vi "main_machine_no_dilution.vi"() -> ()   [LabVIEW 2013]
uses:
  type_defs/robotics_states.ctl
  type_defs/fsc_parameter.ctl
  type_defs/hts_message.ctl
  type_defs/led_mm.ctl
  type_defs/data_message.ctl
  type_defs/reactor.ctl
  type_defs/experiment_states.ctl
  type_defs/global_settings.ctl
  type_defs/mm_states.ctl
  type_defs/experiment_settings.ctl
  type_defs/ps_states.ctl
  hts/type_defs/hts_command_list.ctl
  <vilib>/Utility/file.llb/Write To Spreadsheet File (DBL).vi
  <vilib>/Utility/file.llb/Read From Spreadsheet File (DBL).vi
panel:
  out "GLOBAL STATE":T1
  out "DILUTION  TABLE":dbl[][](array[numeric])
  in  "SETTINGS":T2={"# REACTORS"=8, "17X PORT"=8, "WASTE POSITION "=3, "SECONDS BETWEEN SAMPLING"=600.0, "FACS DIVA DIRECTORY"=path "D:/BDDatabase/BDData", "DATA FILE"=path "C:/Documents and Settings/HES/Desktop/THN20190207_datafile.csv", "REACTORS TO USE"=[5, 4, 7, 6, 11, 12, 2, 1], "PULSE PERIOD"=60, "USE LIGHTS?"=FALSE, "LED FILE"=path "C:/Documents and Settings/HES/Desktop/THN20190207_lightfile.csv", "LED CHANNELS"=[5, 7, 8, 6, 2, 1, 4, 9], "PULSE LENGTH"=60, "SUMMARY FILE"=path "C:/Documents and Settings/HES/Desktop/THN20190207_summaryfile.csv", "OUTGROWTH TIME POINTS"=1.0, "SELECTION VALVE PORT"="COM4", "HTS PORT"="COM6", "DILUTION VOLUME (uL)"=2000, "DILUTION FILE"=path "C:/Documents and Settings/HES/Desktop/THN20190207_dilutionfile.csv", "1X PORT"=10}
  out "EXPERIMENT STATE":T3
  out "TIME TILL SAMPLE":dbl
  out "TIME POINT":i32
  out "SAMPLE #":i32
  out "ITERATION":u32
  out "REACTOR":T5
  out "mAs":dbl[](array[numeric])
  out "NEXT LIGHTS":bool[](array[boolean])
  out "DATA THREAD":T6
  out "LED THREAD":T7
  out "HTS THREAD":T8=enum."DILUTE AND INDUCE"
  out "TIME TILL STROBE":dbl
  in  "Y":T9 items=["DSRED"=30, "TIME"=0, "FSC"=1, "SSC"=6, "FITC"=9]
  in  "X":T9 items=["DSRED"=30, "TIME"=0, "FSC"=1, "SSC"=6, "FITC"=9]
  in  "Reactor to Graph":i32
  out "LOG FITC/SSC":dbl[](graph)
  out "LOG (X/Y)":dynamicdata(graph) caption="Histogram"
  out "Y VERSUS X":T10(graph)
  in  "GRAPH DATA":bool
  in  "REACTOR #":i32
  in  "SHOW REACTOR":bool
  out "CURRENT VALVE":u32
  out "?":timestamp
  out "?":path
  in  "UPDATE STATES":bool
  out "ROBOTICS READY?":T11
  in  "PAUSE":bool
  in  "START EXPERIMENT":bool
  in  "FIND FCS FILE":bool
  in  "INITIALIZE INSTRUMENT":bool
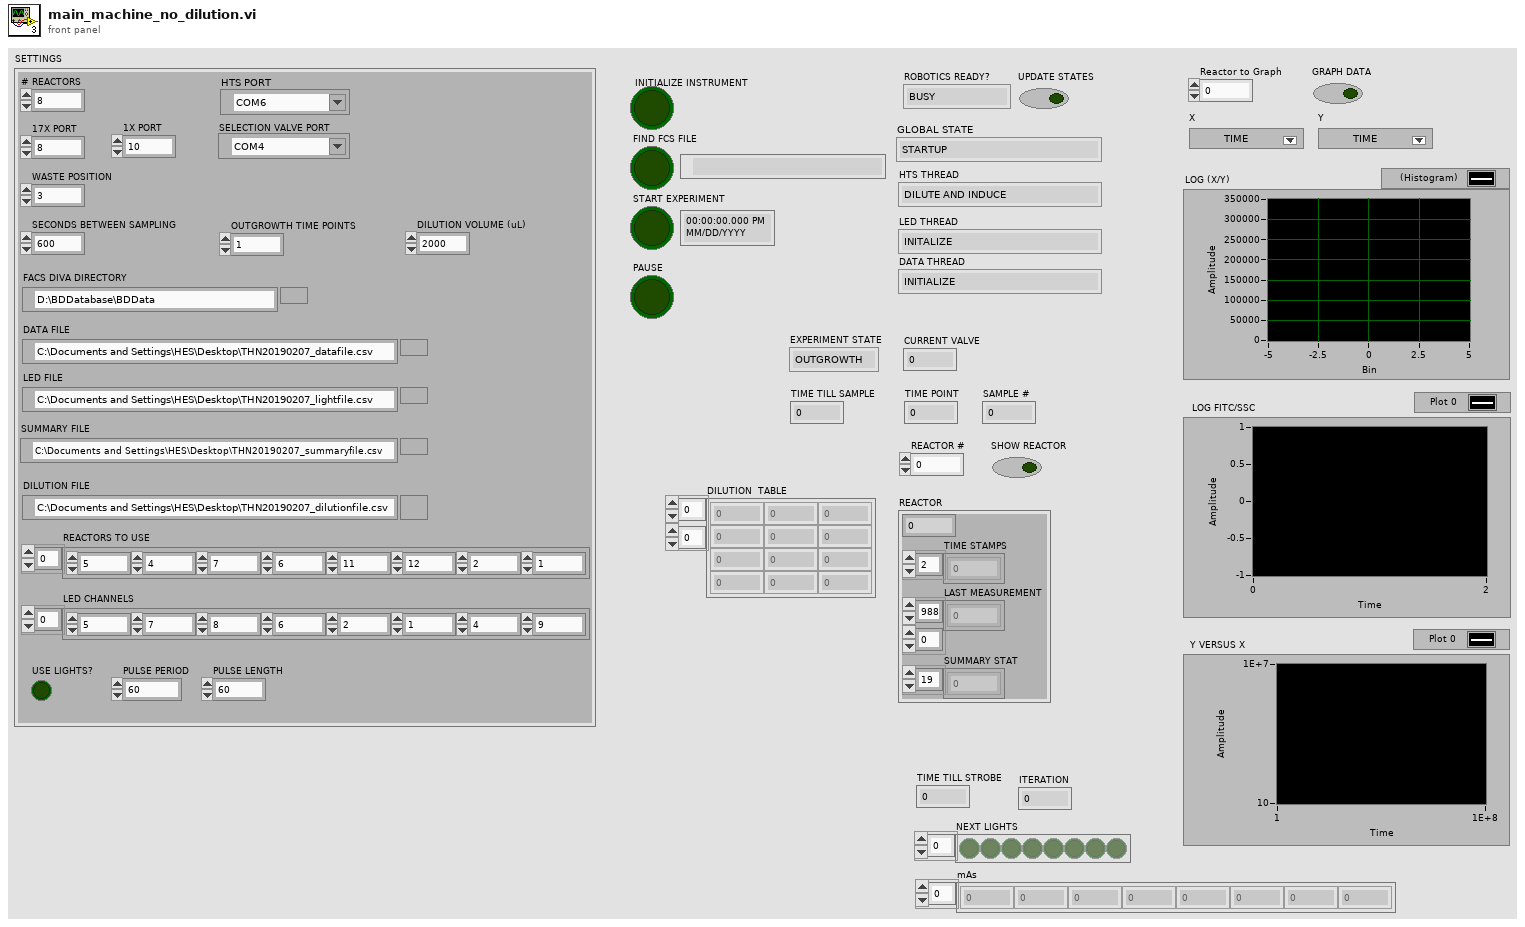
[diagram p1: front panel]
types:
  T1 = typedef "mm_states.ctl" = enum16{"STARTUP", "WAIT FOR COMMAND", "INITIALIZE INSTRUMENT", "FIND FCS FILE ", "START EXPERIMENT", "WAIT TO SAMPLE ", "DILUTE", "TAKE SAMPLE ", "EXIT"}
  T2 = typedef "global_settings.ctl" = cluster{"# REACTORS":u32, "17X PORT":i32, "WASTE POSITION ":i32, "SECONDS BETWEEN SAMPLING":dbl, "FACS DIVA DIRECTORY":path, "DATA FILE":path, "REACTORS TO USE":u32[], "PULSE PERIOD":i32, "USE LIGHTS?":bool, "LED FILE":path, "LED CHANNELS":u32[], "PULSE LENGTH":i32, "SUMMARY FILE":path, "OUTGROWTH TIME POINTS":dbl, "SELECTION VALVE PORT":refnum<visa-resource-name>, "HTS PORT":refnum<visa-resource-name>, "DILUTION VOLUME (uL)":i32, "DILUTION FILE":path, "1X PORT":i32}
  T3 = typedef "experiment_states.ctl" = enum16{"OUTGROWTH", "INDUCTION", "EXPERIMENT"}
  T4 = typedef "reactor.ctl" = dbl
  T5 = cluster{i32, "TIME STAMPS":dbl[], "LAST MEASUREMENT":T4[][], "SUMMARY STAT":dbl[]}
  T6 = typedef "data_message.ctl" = enum16{"INITIALIZE", "UPDATE DATA", "THROW AWAY DATA", "ANALYZE DATA", "SAVE DATA", "SHUTDOWN"}
  T7 = typedef "led_mm.ctl" = enum16{"INITALIZE", "START LEDS", "STROBE", "SHUTDOWN"}
  T8 = typedef "hts_message.ctl" = enum16{"INITIALIZE", "REMOVE CULTURE", "DILUTE AND INDUCE", "SAMPLE REACTOR", "CLEAR LINES", "MOVE TO NEXT", "SHUTDOWN"}
  T9 = typedef "fsc_parameter.ctl" = u16
  T10 = cluster{"LAST MEASUREMENT":dbl[], "LAST MEASUREMENT":dbl[]}
  T11 = typedef "robotics_states.ctl" = enum16{"BUSY", "READY"}
  T12 = typedef "experiment_settings.ctl" = cluster{"fcs file byte offset":i64, "LED Device Handle Out":u32, "START TIME":timestamp, "CURRENT VALVE":u32, "SAMPLE #":i32, "FCS FILE PATH":path, "TIME POINT":i32, "STATE":T3, "TIME TILL SAMPLE":dbl, "DILUTION  TABLE":dbl[][]}
  T13 = cluster{i32, "LED CONTROLS":dbl[], "TIME STAMPS":dbl[], "LAST MEASUREMENT":T4[][], "SUMMARY STAT":dbl[]}
  T14 = typedef "reactors.ctl" = cluster{i32, "TIME STAMPS":dbl[], "LAST MEASUREMENT":T4[][], "SUMMARY STAT":dbl[]}[]
  T15 = typedef "hts_command_list.ctl" = enum16{"INITIALIZE", "ADD MEDIA", "ADD INDUCER", "REMOVE CULTURE", "SAMPLE REACTOR", "CLEAR LINE TO VALVE", "CLEAR LINE TO CYTOMETER", "SAMPLE REACTOR NO DILUTION"}
  T16 = cluster{"LAST MEASUREMENT":T4[], "LAST MEASUREMENT":T4[]}
  T17 = typedef "ps_states.ctl" = enum16{"TAKE OUTGROWTH SAMPLE", "STARTUP", "WAIT FOR COMMAND", "INITIALIZE INSTRUMENT", "FIND FCS FILE ", "START EXPERIMENT", "INDUCE", "WAIT TO SAMPLE ", "TAKE SAMPLE ", "EXIT"}
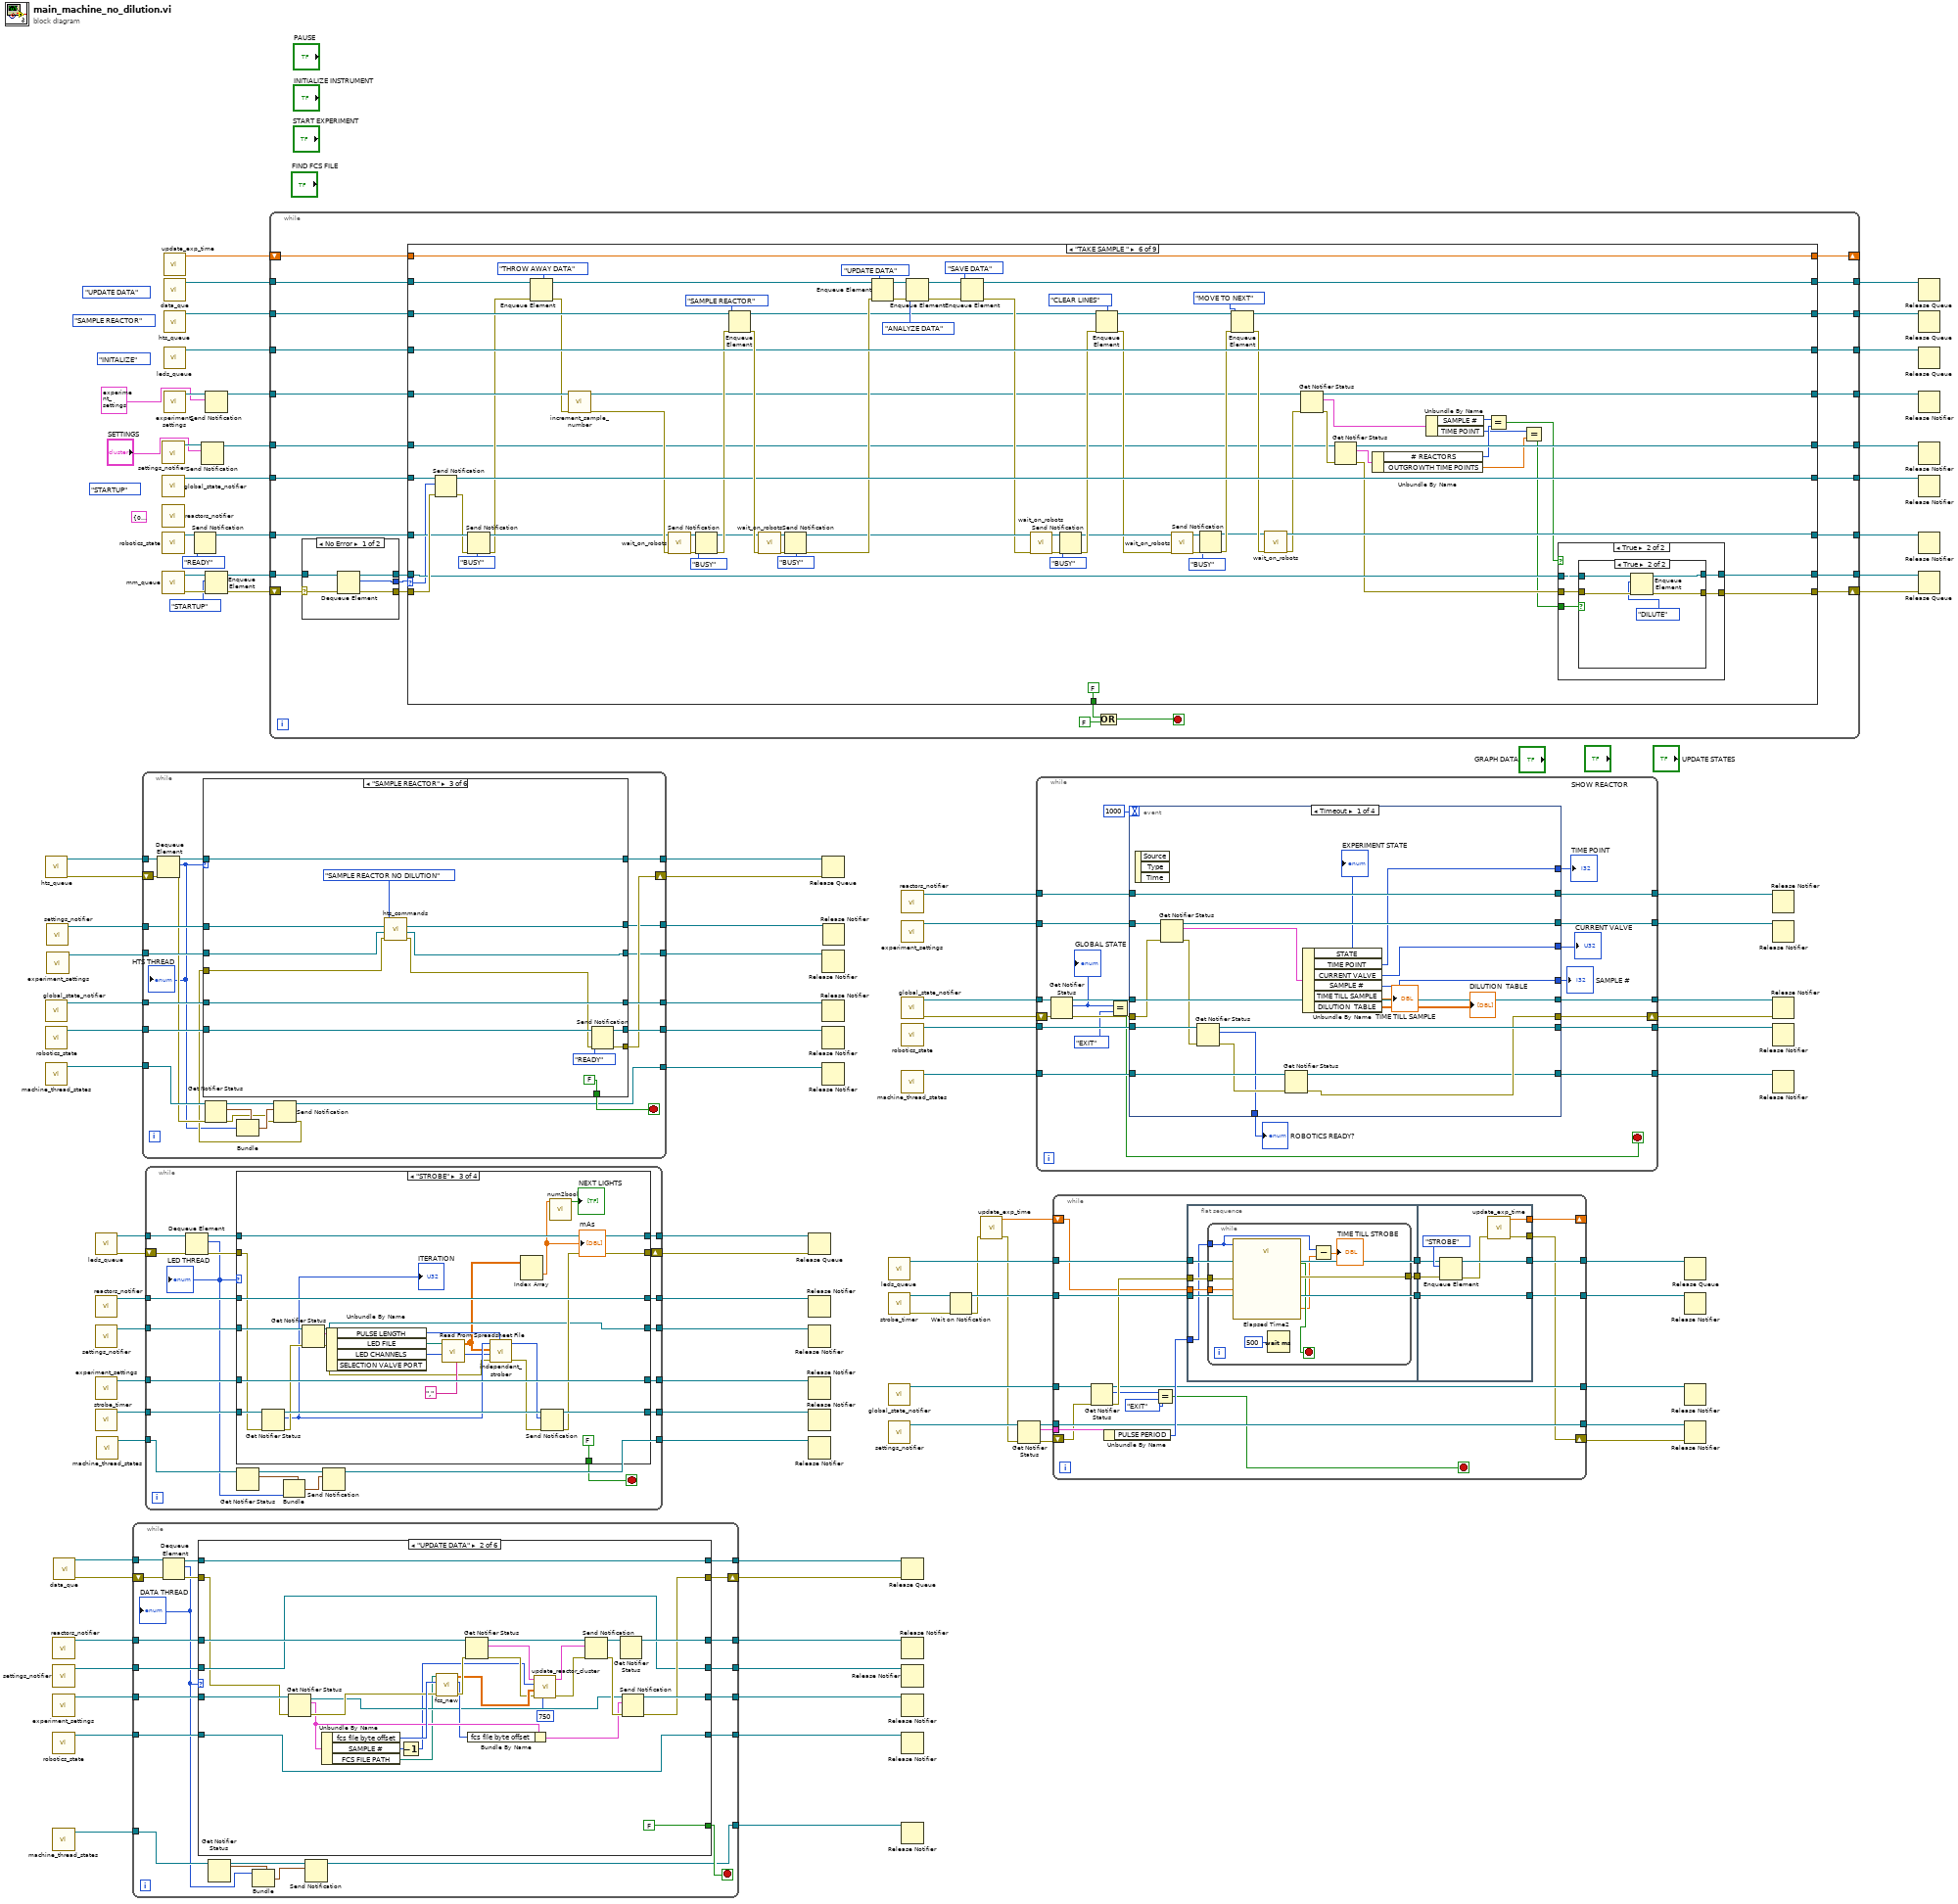
[diagram p0: block diagram]
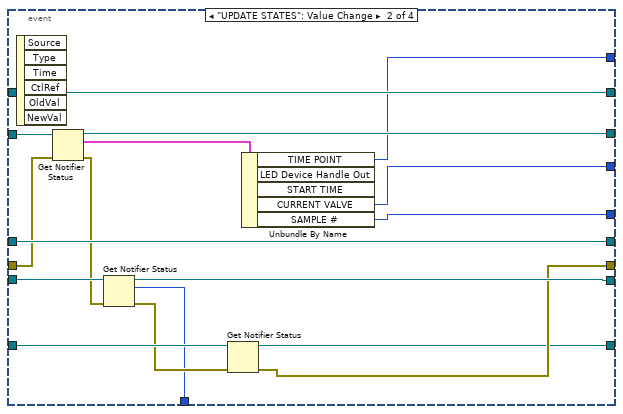
[diagram p2: hidden frame]
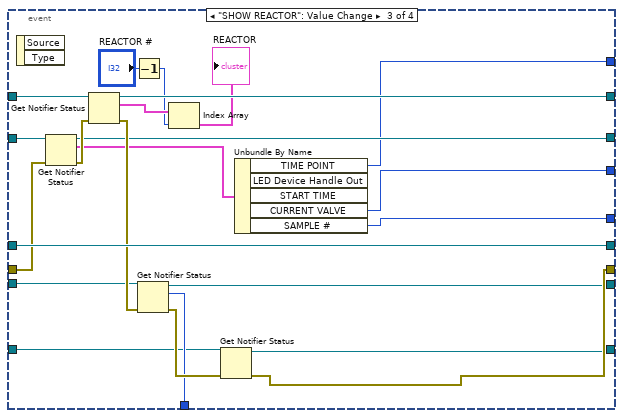
[diagram p3: hidden frame]
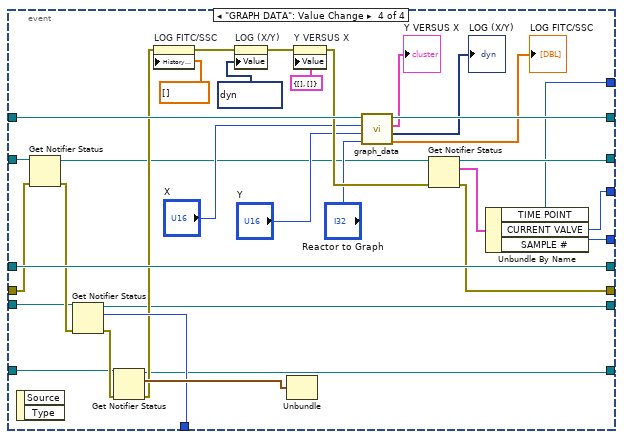
[diagram p4: hidden frame]
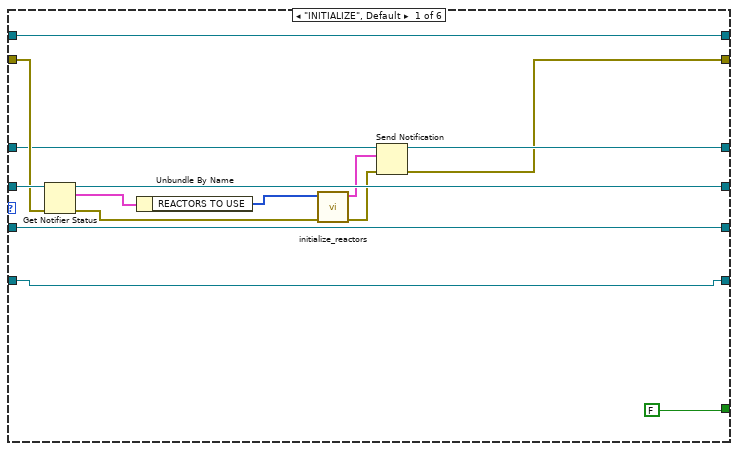
[diagram p5: hidden frame]
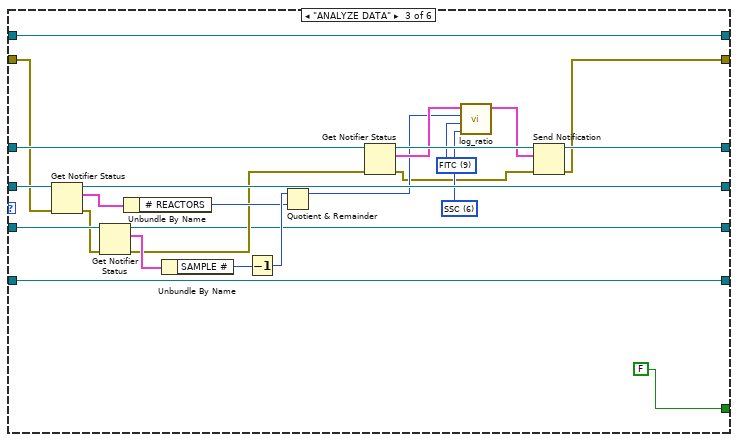
[diagram p6: hidden frame]
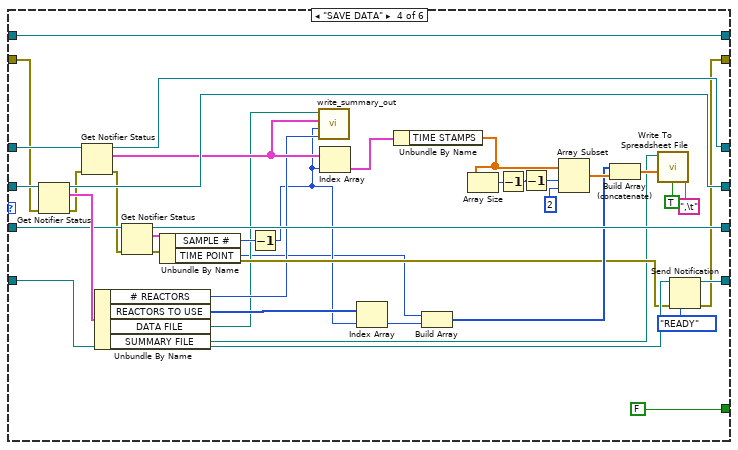
[diagram p7: hidden frame]
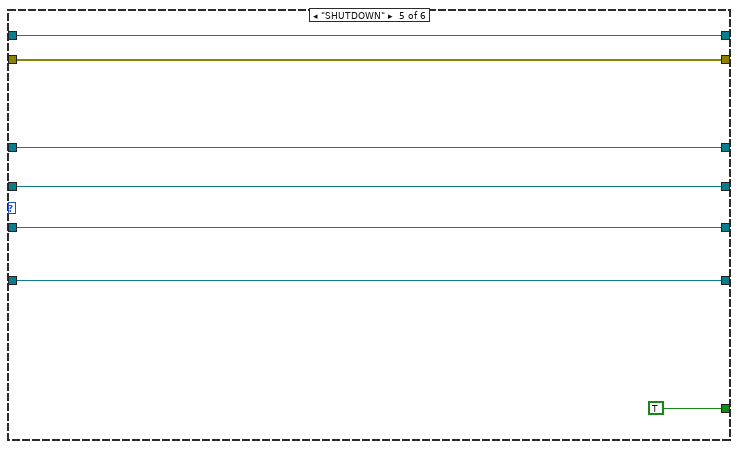
[diagram p8: hidden frame]
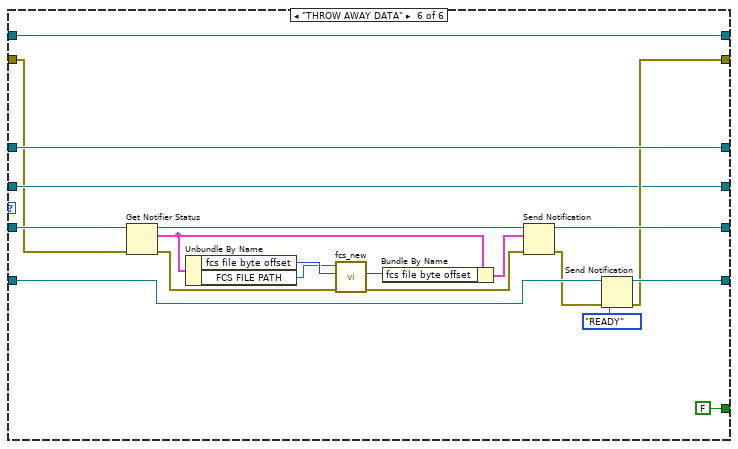
[diagram p9: hidden frame]
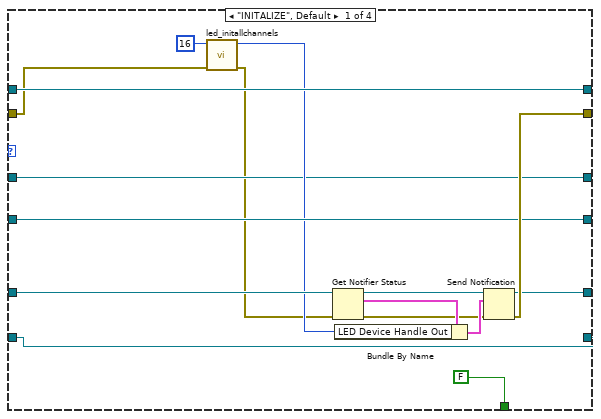
[diagram p10: hidden frame]
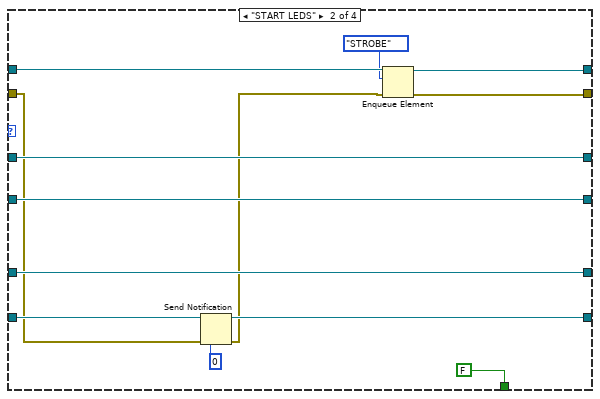
[diagram p11: hidden frame]
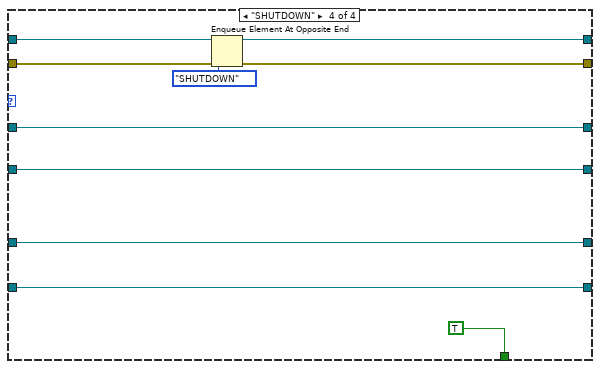
[diagram p12: hidden frame]
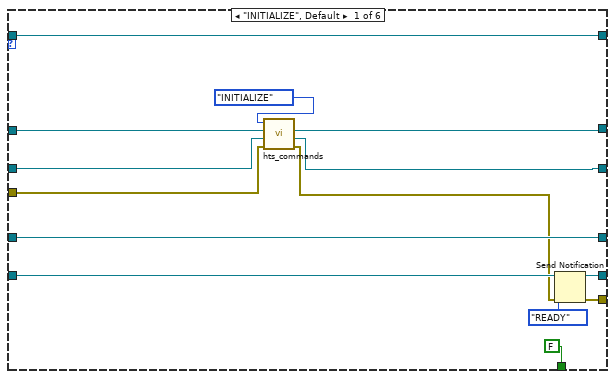
[diagram p13: hidden frame]
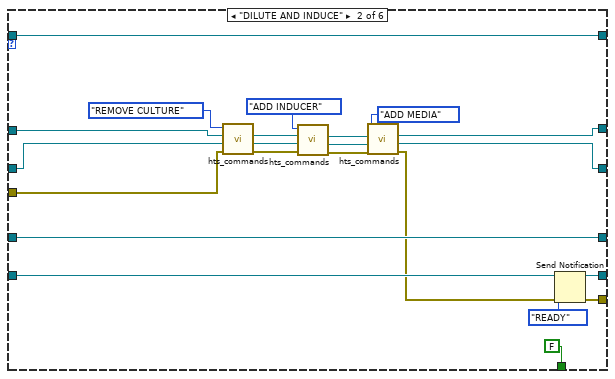
[diagram p14: hidden frame]
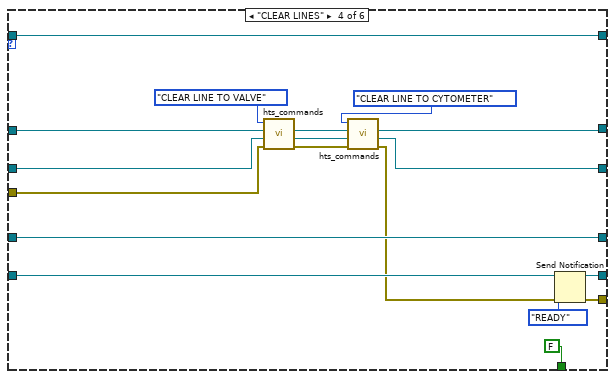
[diagram p15: hidden frame]
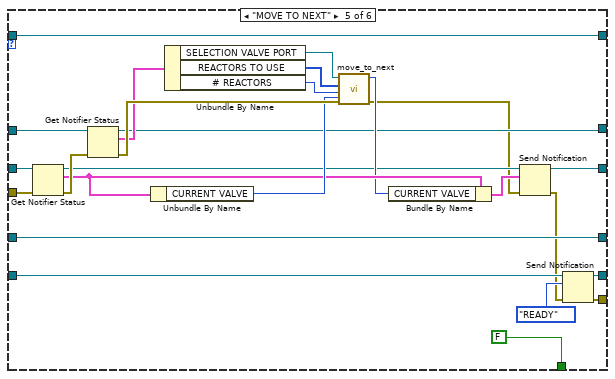
[diagram p16: hidden frame]
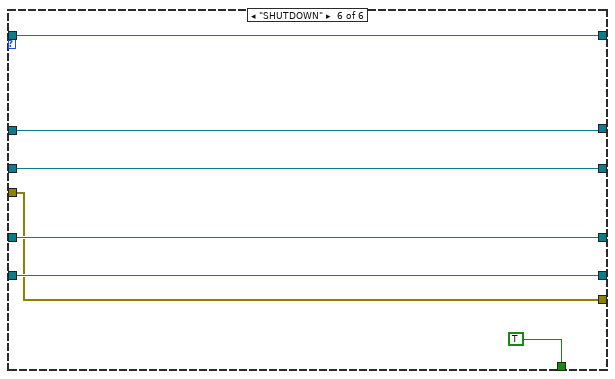
[diagram p17: hidden frame]
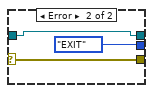
[diagram p18: hidden frame]
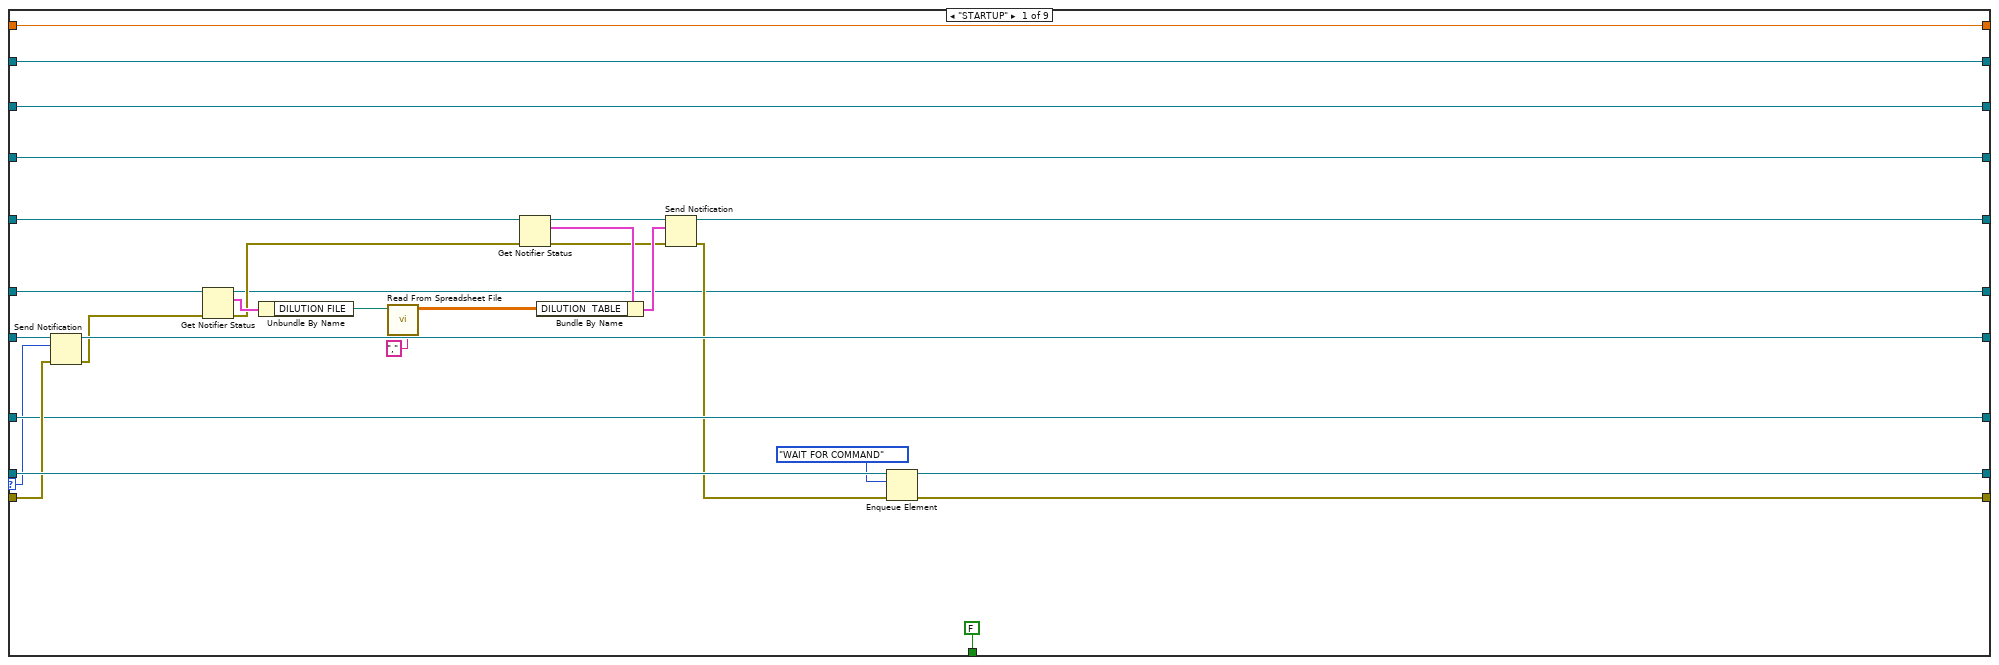
[diagram p19: hidden frame]
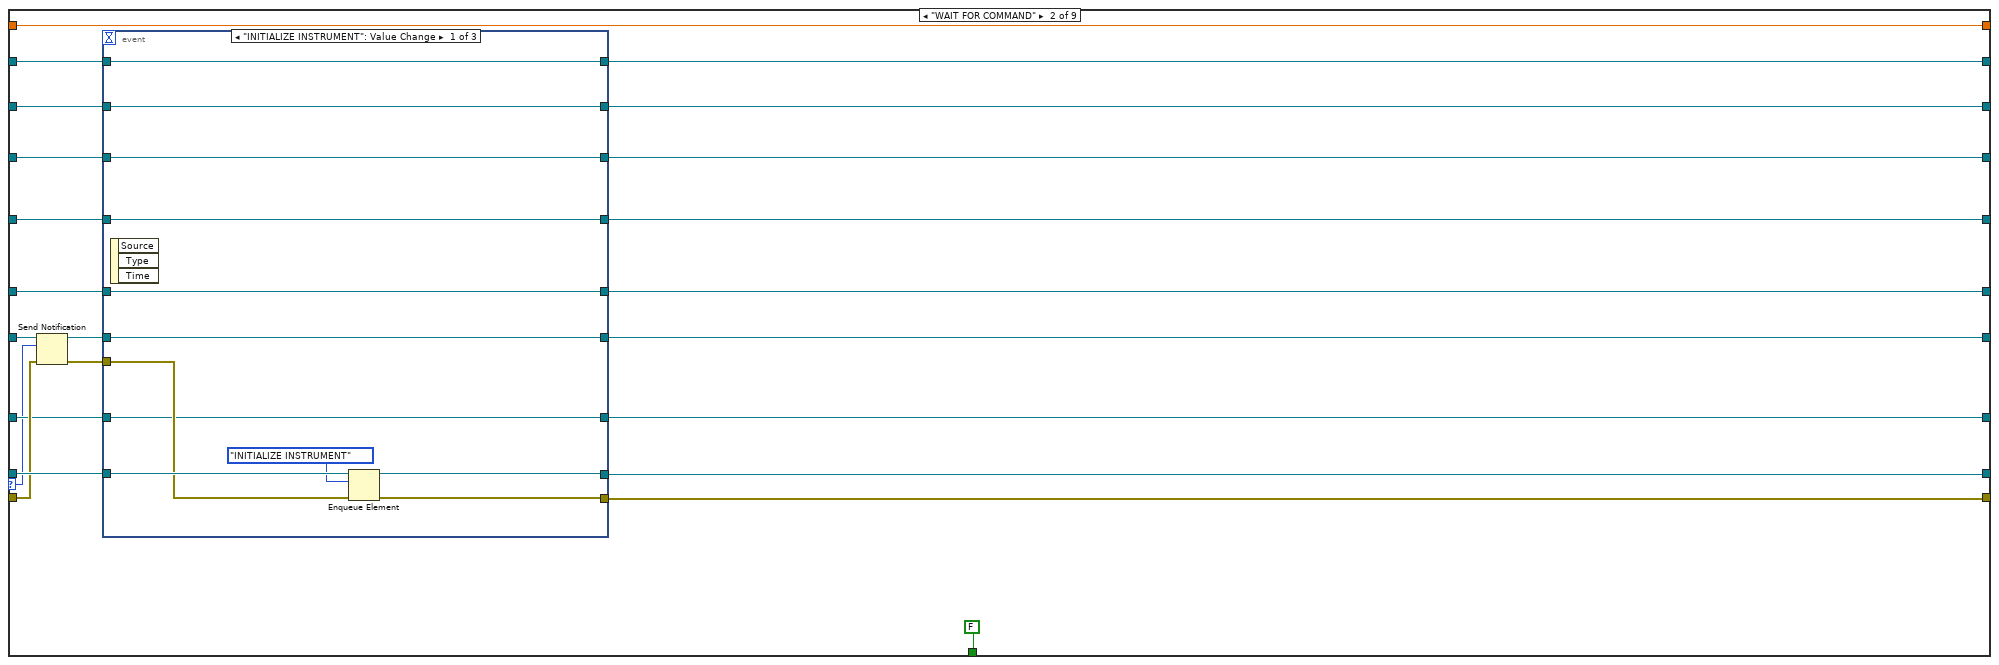
[diagram p20: hidden frame]
diagram:
  (unwired) mm_states."STARTUP" ("element")
  (unwired) T13 {0, "LED CONTROLS"=[], "TIME STAMPS"=[], "LAST MEASUREMENT"=[], "SUMMARY STAT"=[]}
  (unwired) data_message."UPDATE DATA"
  (unwired) led_mm."INITALIZE"
  (unwired) hts_message."SAMPLE REACTOR" ("COMMAND")
  n1 = call "hts_queue.vi"() -> ("error out"=w84:errorcluster, "Queue out"=w85:refnum<queue>)  [unwired: 10 in]
  n2 = call "global_state_notifier.vi"() -> ("GLOBAL STATE"=w78:refnum<notifier>)  [unwired: 10 in, 1 out]
  n3 = call "robotics_state.vi"() -> ("Notifier out"=w72:refnum<notifier>)  [unwired: 10 in, 1 out]
  n4 = call "machine_thread_states.vi"() -> ("Notifier out"=w32:refnum<notifier>)  [unwired: 10 in, 1 out]
  n5 = call "settings_notifier.vi"() -> ("GLOBAL SETTINGS"=w5:refnum<notifier>)  [unwired: 10 in, 1 out]
  n6 = call "experiment_settings.vi"() -> ("Notifier out"=w4:refnum<notifier>)  [unwired: 10 in, 1 out]
  n7 = call "reactors_notifier.vi"() -> ("Notifier out"=w58:refnum<notifier>)  [unwired: 10 in, 1 out]
  n8 = call "settings_notifier.vi"() -> ("GLOBAL SETTINGS"=w57:refnum<notifier>)  [unwired: 10 in, 1 out]
  n9 = call "experiment_settings.vi"() -> ("Notifier out"=w54:refnum<notifier>)  [unwired: 10 in, 1 out]
  n10 = call "robotics_state.vi"() -> ("Notifier out"=w34:refnum<notifier>)  [unwired: 10 in, 1 out]
  n11 = call "machine_thread_states.vi"() -> ("Notifier out"=w28:refnum<notifier>)  [unwired: 10 in, 1 out]
  n12 = call "data_que.vi"() -> ("error out"=w61:errorcluster, "DATA_QUEUE"=w62:refnum<queue>)  [unwired: 10 in]
  n13 = call "leds_queue.vi"() -> ("error out"=w79:errorcluster, "queue out"=w80:refnum<queue>)  [unwired: 10 in]
  n14 = call "reactors_notifier.vi"() -> ("Notifier out"=w49:refnum<notifier>)  [unwired: 10 in, 1 out]
  n15 = call "settings_notifier.vi"() -> ("GLOBAL SETTINGS"=w69:refnum<notifier>)  [unwired: 10 in, 1 out]
  n16 = call "experiment_settings.vi"() -> ("Notifier out"=w65:refnum<notifier>)  [unwired: 10 in, 1 out]
  n17 = call "strobe_timer.vi"() -> ("notifier out"=w46:refnum<notifier>)  [unwired: 10 in, 1 out]
  n18 = call "machine_thread_states.vi"() -> ("Notifier out"=w30:refnum<notifier>)  [unwired: 10 in, 1 out]
  n19 = while {
    tunnel: w62 -> [w120]
    tunnel: [w115] -> w59
    tunnel: w58 -> [w114]
    tunnel: w57 -> [w113]
    tunnel: [w112] -> w56
    tunnel: [w111] -> w55
    tunnel: w54 -> [w110]
    tunnel: [w109] -> w53
    tunnel: w34 -> [w107]
    tunnel: [w106] -> w33
    tunnel: w28 -> [w105]
    tunnel: [w102] -> w27
    shift-right: [w116] -> w60
    shift-left: w61 -> [w118]
    stop <- w108 stop-if-true
    n20 = Dequeue Element(queue=w120, error in (no error)=w118) -> (queue out=w119:refnum<queue>, element=w101:T6, error out=w117:errorcluster)  [unwired: 1 in, 1 out]
    "DATA THREAD" <- w101
    n21 = case shown="\"UPDATE DATA\"" w101 {
      tunnel: w119 -> [w125 w164 w182 w216 w233 w245]
      tunnel: [w127 w141 w166 w197 w232 w238] -> w116
      tunnel: w117 -> [w134 w136 w187 w224 w232 w235]
      tunnel: [w125 w164 w182 w216 w233 w245] -> w115
      tunnel: w114 -> [w130 w159 w189 w225 w231 w244]
      tunnel: w113 -> [w135 w137 w188 w227 w230 w236]
      tunnel: [w131 w137 w183 w213 w230 w236] -> w112
      tunnel: [w128 w142 w184 w214 w231 w244] -> w111
      tunnel: w110 -> [w124 w163 w178 w211 w229 w254]
      tunnel: [w124 w150 w170 w207 w229 w246] -> w109
      tunnel: [FALSE FALSE FALSE FALSE TRUE FALSE] -> w108
      tunnel: w107 -> [w121 w140 w167 w201 w228 w241]
      tunnel: [w121 w140 w167 w200 w228 w240] -> w106
      frame "INITIALIZE", Default {
        n22 = Get Notifier Status(notifier=w135, error in (no error)=w134) -> (notifier out=w131:refnum<notifier>, current notification=w133:T2, error out=w132:errorcluster)  [unwired: 2 out]
        n23 = Unbundle By Name(w133) -> ("REACTORS TO USE"=w122:u32[])
        n24 = call "initialize_reactors.vi"("ERROR IN"=w132, "REACTORS TO USE"=w122) -> ("ERROR OUT"=w129:errorcluster, "REACTORS"=w126:T14)  [unwired: 8 in]
        n25 = Send Notification(notification=w126, notifier=w130, error in (no error)=w129) -> (notifier out=w128:refnum<notifier>, error out=w127:errorcluster)
      }
      frame "UPDATE DATA" {
        n26 = Get Notifier Status(notifier=w163, error in (no error)=w136) -> (notifier out=w151:refnum<notifier>, current notification=w154:T12, error out=w161:errorcluster)  [unwired: 2 out]
        n27 = Unbundle By Name(w154) -> ("fcs file byte offset"=w162:i64, "SAMPLE #"=w148:i32, "FCS FILE PATH"=w147:path)
        n28 = Decrement(x=w148) -> (x-1=w138:i32)
        n29 = call "fcs_new.vi"("error in (no error)"=w161, "byte offset in"=w162, "Path in"=w147) -> ("error out"=w160:errorcluster, "byte offset out"=w153:i64, "new data"=w157:sgl[][])  [unwired: 6 in]
        n30 = Get Notifier Status(notifier=w159, error in (no error)=w160) -> (notifier out=w146:refnum<notifier>, current notification=w158:T14, error out=w145:errorcluster)  [unwired: 2 out]
        n31 = Bundle By Name(cluster=w154, "fcs file byte offset"=w153) -> (w152:T12)
        n32 = call "update_reactor_cluster.vi"("THROW OUT EVENTS"=750, "error in"=w145, "NEW DATA"=w157, "Reactor to update (INDEX)"=w138, "REACTORS"=w158) -> ("error out"=w156:errorcluster, "UPDATED REACTORS"=w144:T14)  [unwired: 5 in]
        n33 = Send Notification(notification=w144, notifier=w146, error in (no error)=w156) -> (notifier out=w143:refnum<notifier>, error out=w155:errorcluster)
        n34 = Get Notifier Status(notifier=w143) -> (notifier out=w142:refnum<notifier>)  [unwired: 1 in, 4 out]
        n35 = Send Notification(notification=w152, notifier=w151, error in (no error)=w155) -> (notifier out=w150:refnum<notifier>, error out=w141:errorcluster)
      }
      frame "ANALYZE DATA" {
        w168 = T9 6 items=["DSRED"=30, "TIME"=0, "FSC"=1, "SSC"=6, "FITC"=9] ("X y")
        w169 = T9 9 items=["DSRED"=30, "TIME"=0, "FSC"=1, "SSC"=6, "FITC"=9] ("X 2")
        n36 = Get Notifier Status(notifier=w188, error in (no error)=w187) -> (notifier out=w183:refnum<notifier>, current notification=w186:T2, error out=w177:errorcluster)  [unwired: 2 out]
        n37 = Get Notifier Status(notifier=w178, error in (no error)=w177) -> (notifier out=w170:refnum<notifier>, current notification=w176:T12, error out=w171:errorcluster)  [unwired: 2 out]
        n38 = Unbundle By Name(w186) -> ("# REACTORS"=w173:u32)
        n39 = Unbundle By Name(w176) -> ("SAMPLE #"=w175:i32)
        n40 = Decrement(x=w175) -> (x-1=w174:i32)
        n41 = Quotient & Remainder(x=w174, y=w173) -> (x-y*floor(x/y)=w172:u32)  [unwired: 1 out]
        n42 = Get Notifier Status(notifier=w189, error in (no error)=w171) -> (notifier out=w185:refnum<notifier>, current notification=w181:T14, error out=w165:errorcluster)  [unwired: 2 out]
        n43 = call "log_ratio.vi"("Y"=w168, "X"=w169, "Reactor (INDEX)"=w172, "REACTORS"=w181) -> ("Updated Reactors"=w180:T14)  [unwired: 5 in, 2 out]
        n44 = Send Notification(notification=w180, notifier=w185, error in (no error)=w165) -> (notifier out=w184:refnum<notifier>, error out=w166:errorcluster)
      }
      frame "SAVE DATA" {
        n45 = Get Notifier Status(notifier=w227, error in (no error)=w224) -> (notifier out=w213:refnum<notifier>, current notification=w226:T2, error out=w210:errorcluster)  [unwired: 2 out]
        n46 = Get Notifier Status(notifier=w225, error in (no error)=w210) -> (notifier out=w214:refnum<notifier>, current notification=w195:T14, error out=w209:errorcluster)  [unwired: 2 out]
        n47 = Unbundle By Name(w226) -> ("# REACTORS"=w194:u32, "REACTORS TO USE"=w205:u32[], "DATA FILE"=w193:path, "SUMMARY FILE"=w192:path)
        n48 = Get Notifier Status(notifier=w211, error in (no error)=w209) -> (notifier out=w207:refnum<notifier>, current notification=w208:T12, error out=w198:errorcluster)  [unwired: 2 out]
        n49 = Unbundle By Name(w208) -> ("SAMPLE #"=w206:i32, "TIME POINT"=w190:i32)
        n50 = Decrement(x=w206) -> (x-1=w191:i32)
        n51 = call "write_summary_out.vi"("# REACTORS"=w194, "REACTOR INDEX"=w191, "REACTOR ARRAY"=w195, "DATA FILE"=w193) -> ()  [unwired: 8 in]
        n52 = Index Array(array=w195, index=w191) -> (element=w223:T5)
        n53 = Index Array(array=w205, index=w191) -> (element=w204:u32)
        n54 = Unbundle By Name(w223) -> ("TIME STAMPS"=w219:dbl[])
        n55 = Build Array(w190, w204) -> (w203:u32[])
        n56 = Array Size(array=w219) -> (size(s)=w221:i32)
        n57 = Decrement(x=w221) -> (x-1=w220:i32)
        n58 = Decrement(x=w220) -> (x-1=w218:i32)
        n59 = Array Subset(array=w219, index=w218, length=2) -> (w215:dbl[])
        n60 = Build Array (concatenate)(w203, w215) -> (w202:dbl[])
        n61 = call-poly <vilib>:"Write To Spreadsheet File.vi"("delimiter (\\t)"=",\t" ("delimiter (\\t)"), "append to file? (new file:F)"=TRUE, "1D data"=w202, "file path (dialog if empty)"=w192) -> ()  [unwired: 4 in, 1 out]
        n62 = Send Notification(notification=robotics_states."READY", notifier=w201, error in (no error)=w198) -> (notifier out=w200:refnum<notifier>, error out=w197:errorcluster)
      }
      frame "SHUTDOWN" {
      }
      frame "THROW AWAY DATA" {
        n63 = Get Notifier Status(notifier=w254, error in (no error)=w235) -> (notifier out=w251:refnum<notifier>, current notification=w249:T12, error out=w253:errorcluster)  [unwired: 2 out]
        n64 = Unbundle By Name(w249) -> ("fcs file byte offset"=w252:i64, "FCS FILE PATH"=w242:path)
        n65 = call "fcs_new.vi"("error in (no error)"=w253, "byte offset in"=w252, "Path in"=w242) -> ("error out"=w250:errorcluster, "byte offset out"=w248:i64)  [unwired: 6 in, 1 out]
        n66 = Bundle By Name(cluster=w249, "fcs file byte offset"=w248) -> (w247:T12)
        n67 = Send Notification(notification=w247, notifier=w251, error in (no error)=w250) -> (notifier out=w246:refnum<notifier>, error out=w239:errorcluster)
        n68 = Send Notification(notification=robotics_states."READY", notifier=w241, error in (no error)=w239) -> (notifier out=w240:refnum<notifier>, error out=w238:errorcluster)
      }
    }
    n69 = Get Notifier Status(notifier=w105) -> (notifier out=w103:refnum<notifier>, current notification=w104:cluster{T6, "COMMAND":T8, T7})  [unwired: 1 in, 3 out]
    n70 = Bundle(cluster=w104, w101) -> (w100:cluster{T6, "COMMAND":T8, T7})  [unwired: 2 in]
    n71 = Send Notification(notification=w100, notifier=w103) -> (notifier out=w102:refnum<notifier>)  [unwired: 1 in, 1 out]
  }
  n72 = while {
    tunnel: w85 -> [w277]
    tunnel: [w274] -> w83
    tunnel: w4 -> [w273]
    tunnel: w78 -> [w272]
    tunnel: [w271] -> w73
    tunnel: w72 -> [w270]
    tunnel: [w269] -> w71
    shift-right: [w268] -> w70
    shift-left: w84 -> [w276]
    tunnel: w5 -> [w267]
    tunnel: [w266] -> w52
    tunnel: [w265] -> w51
    tunnel: w32 -> [w263]
    tunnel: [w260] -> w31
    stop <- w264 stop-if-true
    n73 = Dequeue Element(queue=w277, error in (no error)=w276) -> (queue out=w275:refnum<queue>, element=w255:T8, error out=w258:errorcluster)  [unwired: 1 in, 1 out]
    "HTS THREAD" <- w255
    n74 = Get Notifier Status(notifier=w263, error in (no error)=w258) -> (notifier out=w262:refnum<notifier>, current notification=w259:cluster{T6, "COMMAND":T8, T7}, error out=w257:errorcluster)  [unwired: 2 out]
    n75 = Bundle(cluster=w259, "COMMAND"=w255) -> (w261:cluster{T6, "COMMAND":T8, T7})  [unwired: 2 in]
    n76 = Send Notification(notification=w261, notifier=w262, error in (no error)=w257) -> (notifier out=w260:refnum<notifier>, error out=w256:errorcluster)
    n77 = case shown="\"SAMPLE REACTOR\"" w255 {
      tunnel: w275 -> [w291 w313 w327 w345 w367 w376]
      tunnel: [w291 w313 w327 w345 w367 w376] -> w274
      tunnel: w273 -> [w284 w295 w320 w338 w370 w375]
      tunnel: w272 -> [w290 w312 w326 w344 w368 w374]
      tunnel: [w290 w312 w326 w344 w368 w374] -> w271
      tunnel: w270 -> [w289 w311 w325 w343 w363 w373]
      tunnel: [w288 w310 w324 w342 w369 w373] -> w269
      tunnel: [w287 w309 w323 w341 w360 w372] -> w268
      tunnel: w267 -> [w279 w296 w315 w336 w365 w371]
      tunnel: [w283 w297 w319 w331 w348 w371] -> w266
      tunnel: [w282 w292 w318 w332 w349 w375] -> w265
      tunnel: [FALSE FALSE FALSE FALSE FALSE TRUE] -> w264
      tunnel: w256 -> [w281 w294 w317 w337 w359 w372]
      frame "INITIALIZE", Default {
        n78 = call "hts_commands.vi"("Error IN"=w281, "EXP SETTINGS"=w284, "SETTINGS"=w279, "COMMAND"=hts_command_list."INITIALIZE") -> ("error out"=w280:errorcluster, "EXP Settings"=w282:refnum<notifier>, "Settings"=w283:refnum<notifier>)  [unwired: 5 in]
        n79 = Send Notification(notification=robotics_states."READY", notifier=w289, error in (no error)=w280) -> (notifier out=w288:refnum<notifier>, error out=w287:errorcluster)
      }
      frame "DILUTE AND INDUCE" {
        n80 = call "hts_commands.vi"("Error IN"=w294, "EXP SETTINGS"=w295, "SETTINGS"=w296, "COMMAND"=hts_command_list."REMOVE CULTURE") -> ("error out"=w301:errorcluster, "EXP Settings"=w305:refnum<notifier>, "Settings"=w306:refnum<notifier>)  [unwired: 5 in]
        n81 = call "hts_commands.vi"("Error IN"=w301, "EXP SETTINGS"=w305, "SETTINGS"=w306, "COMMAND"=hts_command_list."ADD INDUCER") -> ("error out"=w300:errorcluster, "EXP Settings"=w304:refnum<notifier>, "Settings"=w303:refnum<notifier>)  [unwired: 5 in]
        n82 = call "hts_commands.vi"("Error IN"=w300, "EXP SETTINGS"=w304, "SETTINGS"=w303, "COMMAND"=hts_command_list."ADD MEDIA") -> ("error out"=w293:errorcluster, "EXP Settings"=w292:refnum<notifier>, "Settings"=w297:refnum<notifier>)  [unwired: 5 in]
        n83 = Send Notification(notification=robotics_states."READY", notifier=w311, error in (no error)=w293) -> (notifier out=w310:refnum<notifier>, error out=w309:errorcluster)
      }
      frame "SAMPLE REACTOR" {
        n84 = call "hts_commands.vi"("Error IN"=w317, "EXP SETTINGS"=w320, "SETTINGS"=w315, "COMMAND"=hts_command_list."SAMPLE REACTOR NO DILUTION") -> ("error out"=w316:errorcluster, "EXP Settings"=w318:refnum<notifier>, "Settings"=w319:refnum<notifier>)  [unwired: 5 in]
        n85 = Send Notification(notification=robotics_states."READY", notifier=w325, error in (no error)=w316) -> (notifier out=w324:refnum<notifier>, error out=w323:errorcluster)
      }
      frame "CLEAR LINES" {
        n86 = call "hts_commands.vi"("Error IN"=w337, "EXP SETTINGS"=w338, "SETTINGS"=w336, "COMMAND"=hts_command_list."CLEAR LINE TO VALVE") -> ("error out"=w335:errorcluster, "EXP Settings"=w334:refnum<notifier>, "Settings"=w333:refnum<notifier>)  [unwired: 5 in]
        n87 = call "hts_commands.vi"("Error IN"=w335, "EXP SETTINGS"=w334, "SETTINGS"=w333, "COMMAND"=hts_command_list."CLEAR LINE TO CYTOMETER") -> ("error out"=w330:errorcluster, "EXP Settings"=w332:refnum<notifier>, "Settings"=w331:refnum<notifier>)  [unwired: 5 in]
        n88 = Send Notification(notification=robotics_states."READY", notifier=w343, error in (no error)=w330) -> (notifier out=w342:refnum<notifier>, error out=w341:errorcluster)
      }
      frame "MOVE TO NEXT" {
        n89 = Get Notifier Status(notifier=w370, error in (no error)=w359) -> (notifier out=w350:refnum<notifier>, current notification=w353:T12, error out=w364:errorcluster)  [unwired: 2 out]
        n90 = Get Notifier Status(notifier=w365, error in (no error)=w364) -> (notifier out=w348:refnum<notifier>, current notification=w357:T2, error out=w362:errorcluster)  [unwired: 2 out]
        n91 = Unbundle By Name(w353) -> ("CURRENT VALVE"=w358:u32)
        n92 = Unbundle By Name(w357) -> ("SELECTION VALVE PORT"=w356:refnum<visa-resource-name>, "REACTORS TO USE"=w355:u32[], "# REACTORS"=w354:u32)
        n93 = call "move_to_next.vi"("CURRENT VALVE"=w358, "error in (no error)"=w362, "# REACTORS"=w354, "REACTORS TO USE"=w355, "VISA Refnum in"=w356) -> ("error out"=w347:errorcluster, "New Position"=w352:u32)  [unwired: 5 in]
        n94 = Bundle By Name(cluster=w353, "CURRENT VALVE"=w352) -> (w351:T12)
        n95 = Send Notification(notification=w351, notifier=w350, error in (no error)=w347) -> (notifier out=w349:refnum<notifier>, error out=w346:errorcluster)
        n96 = Send Notification(notification=robotics_states."READY", notifier=w363, error in (no error)=w346) -> (notifier out=w369:refnum<notifier>, error out=w360:errorcluster)
      }
      frame "SHUTDOWN" {
      }
    }
  }
  n97 = while {
    tunnel: w80 -> [w388]
    tunnel: w69 -> [w396]
    tunnel: [w395] -> w68
    tunnel: [w394] -> w67
    shift-right: [w392] -> w66
    shift-left: w79 -> [w387]
    tunnel: w65 -> [w393]
    tunnel: [w391] -> w64
    tunnel: w49 -> [w390]
    tunnel: [w389] -> w48
    tunnel: [w386] -> w47
    tunnel: w46 -> [w385]
    tunnel: w30 -> [w384]
    tunnel: [w381] -> w29
    stop <- w380 stop-if-true
    n98 = Dequeue Element(queue=w388, error in (no error)=w387) -> (queue out=w398:refnum<queue>, element=w379:T7, error out=w397:errorcluster)  [unwired: 1 in, 1 out]
    "LED THREAD" <- w379
    n99 = case shown="\"STROBE\"" w379 {
      tunnel: w398 -> [w414 w419 w451 w457]
      tunnel: w397 -> [w400 w421 w440 w455]
      tunnel: w396 -> [w404 w426 w446 w460]
      tunnel: [w404 w426 w437 w460] -> w395
      tunnel: [w414 w418 w451 w456] -> w394
      tunnel: w393 -> [w413 w427 w448 w459]
      tunnel: [w408 w416 w438 w454] -> w392
      tunnel: [w407 w427 w448 w459] -> w391
      tunnel: w390 -> [w401 w425 w449 w461]
      tunnel: [w401 w425 w449 w461] -> w389
      tunnel: [w406 w423 w443 w458] -> w386
      tunnel: w385 -> [w406 w424 w447 w458]
      tunnel: [FALSE FALSE FALSE TRUE] -> w380
      frame "INITALIZE", Default {
        n100 = call "led_initallchannels.vi"("ERROR"=w400, "Channels"=16) -> ("ERROR OUT"=w399:errorcluster, "Device Handle Out"=w402:u32)  [unwired: 8 in]
        n101 = Get Notifier Status(notifier=w413, error in (no error)=w399) -> (notifier out=w411:refnum<notifier>, current notification=w412:T12, error out=w409:errorcluster)  [unwired: 2 out]
        n102 = Bundle By Name(cluster=w412, "LED Device Handle Out"=w402) -> (w410:T12)
        n103 = Send Notification(notification=w410, notifier=w411, error in (no error)=w409) -> (notifier out=w407:refnum<notifier>, error out=w408:errorcluster)
      }
      frame "START LEDS" {
        n104 = Send Notification(notification=u32 0, notifier=w424, error in (no error)=w421) -> (notifier out=w423:refnum<notifier>, error out=w417:errorcluster)
        n105 = Enqueue Element(queue=w419, element=led_mm."STROBE", error in (no error)=w417) -> (queue out=w418:refnum<queue>, error out=w416:errorcluster)  [unwired: 1 in, 1 out]
      }
      frame "STROBE" {
        n106 = Get Notifier Status(notifier=w447, error in (no error)=w440) -> (notifier out=w444:refnum<notifier>, current notification=w434:u32, error out=w439:errorcluster)  [unwired: 2 out]
        "ITERATION" <- w434
        n107 = Get Notifier Status(notifier=w446, error in (no error)=w439) -> (notifier out=w437:refnum<notifier>, current notification=w445:T2, error out=w430:errorcluster)  [unwired: 2 out]
        n108 = Unbundle By Name(w445) -> ("PULSE LENGTH"=w433:i32, "LED FILE"=w442:path, "LED CHANNELS"=w428:u32[])  [unwired: 1 out]
        n109 = call-poly <vilib>:"Read From Spreadsheet File.vi"("delimiter (\\t)"="," ("delimiter (\\t)"), "file path (dialog if empty)"=w442) -> ("all rows"=w429:dbl[][])  [unwired: 5 in, 4 out]
        n110 = call "independent_strober.vi"("light pulse (s)"=w433, "error in (no error)"=w430, "LED CHANNELS"=w428, "LED_TABLE"=w429, "Iteration in"=w434) -> ("error out"=w431:errorcluster, "Iteration out"=w432:u32)  [unwired: 5 in]
        n111 = Index Array(array=w429) -> (element=w436:dbl[])  [unwired: 2 in]
        "mAs" <- w436
        n112 = Send Notification(notification=w432, notifier=w444, error in (no error)=w431) -> (notifier out=w443:refnum<notifier>, error out=w438:errorcluster)
        n113 = call "num2bool.vi"("INTERGER ARRAY"=w436) -> ("BOOLEAN ARRAY"=→"NEXT LIGHTS":bool[])  [unwired: 10 in]
      }
      frame "SHUTDOWN" {
        n114 = Enqueue Element At Opposite End(queue=w457, element=led_mm."SHUTDOWN", error in (no error)=w455) -> (queue out=w456:refnum<queue>, error out=w454:errorcluster)  [unwired: 1 in, 1 out]
      }
    }
    n115 = Get Notifier Status(notifier=w384) -> (notifier out=w382:refnum<notifier>, current notification=w383:cluster{T6, "COMMAND":T8, T7})  [unwired: 1 in, 3 out]
    n116 = Bundle(cluster=w383, w379) -> (w378:cluster{T6, "COMMAND":T8, T7})  [unwired: 2 in]
    n117 = Send Notification(notification=w378, notifier=w382) -> (notifier out=w381:refnum<notifier>)  [unwired: 1 in, 1 out]
  }
  n118 = call "settings_notifier.vi"() -> ("GLOBAL SETTINGS"=w82:refnum<notifier>)  [unwired: 10 in, 1 out]
  n119 = call "global_state_notifier.vi"() -> ("GLOBAL STATE"=w93:refnum<notifier>)  [unwired: 10 in, 1 out]
  n120 = call "reactors_notifier.vi"() -> ()  [unwired: 10 in, 2 out]
  n121 = call "robotics_state.vi"() -> ("Notifier out"=w77:refnum<notifier>)  [unwired: 10 in, 1 out]
  n122 = call "mm_queue.vi"() -> ("error out"=w88:errorcluster, "MM_STATE"=w90:refnum<queue>)  [unwired: 10 in]
  n123 = call "update_exp_time.vi"() -> ("double precision float"=w11:dbl)  [unwired: 10 in, 1 out]
  n124 = call "data_que.vi"() -> ("DATA_QUEUE"=w99:refnum<queue>)  [unwired: 10 in, 1 out]
  n125 = call "hts_queue.vi"() -> ("Queue out"=w98:refnum<queue>)  [unwired: 10 in, 1 out]
  n126 = call "leds_queue.vi"() -> ("queue out"=w97:refnum<queue>)  [unwired: 10 in, 1 out]
  n127 = call "experiment_settings.vi"() -> ("Notifier out"=w16:refnum<notifier>)  [unwired: 10 in, 1 out]
  n128 = Send Notification(notification=robotics_states."READY", notifier=w77) -> (notifier out=w76:refnum<notifier>)  [unwired: 1 in, 1 out]
  n129 = Send Notification(notification="SETTINGS", notifier=w82) -> (notifier out=w81:refnum<notifier>)  [unwired: 1 in, 1 out]
  n130 = Send Notification(notification=T12 {"fcs file byte offset"=0, "LED Device Handle Out"=0, "START TIME"=timestamp(0 s since 1904-01-01), "CURRENT VALVE"=0, "SAMPLE #"=0, "FCS FILE PATH"=path "", "TIME POINT"=0, "STATE"=enum."OUTGROWTH", "TIME TILL SAMPLE"=0.0, "DILUTION  TABLE"=[]} ("EXPERIMENT SETTINGS"), notifier=w16) -> (notifier out=w15:refnum<notifier>)  [unwired: 1 in, 1 out]
  n131 = Enqueue Element(queue=w90, element=mm_states."STARTUP", error in (no error)=w88) -> (queue out=w89:refnum<queue>, error out=w87:errorcluster)  [unwired: 1 in, 1 out]
  n132 = while {
    tunnel: w93 -> [w481]
    tunnel: [w480] -> w92
    tunnel: w89 -> [w478]
    tunnel: [w474] -> w91
    tunnel: w81 -> [w471]
    tunnel: w99 -> [w487]
    tunnel: [w486] -> w96
    tunnel: w98 -> [w485]
    tunnel: [w484] -> w95
    tunnel: w97 -> [w483]
    tunnel: [w482] -> w94
    shift-right: [w475] -> w86
    shift-left: w87 -> [w479]
    tunnel: w76 -> [w473]
    tunnel: [w472] -> w74
    tunnel: w15 -> [w470]
    tunnel: [w469] -> w63
    tunnel: [w468] -> w50
    shift-right: [w466] -> _
    shift-left: w11 -> [w467]
    stop <- w463 stop-if-true
    n133 = case shown="No Error" w479 {
      selector: w479 -> [w490 w494]
      tunnel: w478 -> [w492 w495]
      tunnel: [w491 w495] -> w477
      tunnel: [w489 w494] -> w476
      tunnel: [w488 mm_states."EXIT" ("Enum")] -> w462
      frame No Error {
        n134 = Dequeue Element(queue=w492, error in (no error)=w490) -> (queue out=w491:refnum<queue>, element=w488:T1, error out=w489:errorcluster)  [unwired: 1 in, 1 out]
      }
      frame Error {
      }
    }
    n135 = case shown="\"TAKE SAMPLE \"" w462 {
      selector: w462 -> [w511 w525 w587 w627 w663 w707 w803 w822 w858]
      tunnel: w487 -> [w524 w541 w607 w633 w679 w746 w811 w838 w871]
      tunnel: [w524 w540 w606 w633 w679 w722 w811 w837 w871] -> w486
      tunnel: w485 -> [w523 w543 w619 w654 w680 w727 w817 w831 w870]
      tunnel: [w523 w542 w617 w654 w680 w736 w798 w830 w870] -> w484
      tunnel: w483 -> [w522 w545 w600 w653 w661 w772 w812 w829 w849]
      tunnel: [w522 w544 w599 w653 w661 w772 w812 w828 w848] -> w482
      tunnel: [w517 w534 w612 w655 w681 w773 w801 w824 w850] -> w480
      tunnel: w481 -> [w518 w539 w616 w657 w686 w776 w802 w836 w880]
      tunnel: w477 -> [w521 w547 w614 w638 w670 w711 w810 w843 w876]
      tunnel: [w520 w546 w613 w637 w669 w712 w808 w843 w872] -> w474
      tunnel: w476 -> [w516 w537 w610 w656 w685 w770 w805 w835 w879]
      tunnel: [w519 w535 w592 w635 w666 w709 w809 w823 w845] -> w475
      tunnel: w473 -> [w515 w533 w611 w634 w682 w743 w819 w842 w869]
      tunnel: [w515 w532 w603 w634 w682 w728 w799 w842 w869] -> w472
      tunnel: w471 -> [w510 w529 w598 w652 w683 w713 w814 w841 w857]
      tunnel: w470 -> [w508 w531 w585 w646 w658 w771 w813 w840 w878]
      tunnel: [w497 w530 w588 w640 w662 w715 w813 w840 w861] -> w469
      tunnel: [w496 w528 w593 w632 w660 w708 w814 w841 w847] -> w468
      tunnel: w467 -> [w514 w527 w602 w631 w671 w769 w821 w844 _]
      tunnel: [w514 w527 w602 w631 w665 w769 w821 w844 w867] -> w466
      tunnel: [FALSE FALSE FALSE FALSE FALSE FALSE FALSE TRUE FALSE] -> w464
      frame "STARTUP" {
        n136 = Send Notification(notification=w511, notifier=w518, error in (no error)=w516) -> (notifier out=w517:refnum<notifier>, error out=w501:errorcluster)
        n137 = Get Notifier Status(notifier=w510, error in (no error)=w501) -> (notifier out=w496:refnum<notifier>, current notification=w509:T2, error out=w500:errorcluster)  [unwired: 2 out]
        n138 = Unbundle By Name(w509) -> ("DILUTION FILE"=w504:path)
        n139 = call-poly <vilib>:"Read From Spreadsheet File.vi"("delimiter (\\t)"="," ("delimiter (\\t)"), "file path (dialog if empty)"=w504) -> ("all rows"=w503:dbl[][])  [unwired: 5 in, 4 out]
        n140 = Get Notifier Status(notifier=w508, error in (no error)=w500) -> (notifier out=w507:refnum<notifier>, current notification=w506:T12, error out=w499:errorcluster)  [unwired: 2 out]
        n141 = Bundle By Name(cluster=w506, "DILUTION  TABLE"=w503) -> (w502:T12)
        n142 = Send Notification(notification=w502, notifier=w507, error in (no error)=w499) -> (notifier out=w497:refnum<notifier>, error out=w498:errorcluster)
        n143 = Enqueue Element(queue=w521, element=mm_states."WAIT FOR COMMAND", error in (no error)=w498) -> (queue out=w520:refnum<queue>, error out=w519:errorcluster)  [unwired: 1 in, 1 out]
      }
      frame "WAIT FOR COMMAND" {
        n144 = Send Notification(notification=w525, notifier=w539, error in (no error)=w537) -> (notifier out=w538:refnum<notifier>, error out=w536:errorcluster)
        n145 = event shown="[0] \"INITIALIZE INSTRUMENT\": Value Change" {
          selector: _ -> [_ _ _]
          dyn-events: _ -> [_ _ _]
          timeout: _ -> [_ _ _]
          tunnel: w547 -> [w559 w571 w583]
          tunnel: [w558 w565 w580] -> w535
          tunnel: [w557 w570 w582] -> w546
          tunnel: w538 -> [w552 w566 w576]
          tunnel: w545 -> [w556 w567 w579]
          tunnel: [w556 w567 w579] -> w544
          tunnel: w543 -> [w555 w568 w578]
          tunnel: [w555 w568 w578] -> w542
          tunnel: w541 -> [w554 w569 w577]
          tunnel: [w554 w569 w577] -> w540
          tunnel: w536 -> [w553 w564 w581]
          tunnel: [w552 w566 w576] -> w534
          tunnel: w533 -> [w551 w563 w575]
          tunnel: [w551 w563 w575] -> w532
          tunnel: w531 -> [w550 w562 w574]
          tunnel: [w550 w562 w574] -> w530
          tunnel: w529 -> [w549 w561 w573]
          tunnel: [w549 w561 w573] -> w528
          event "INITIALIZE INSTRUMENT": Value Change {
            n146 = event-data() -> ()  [unwired: 1 in, 3 out]
            n147 = Enqueue Element(queue=w559, element=mm_states."INITIALIZE INSTRUMENT", error in (no error)=w553) -> (queue out=w557:refnum<queue>, error out=w558:errorcluster)  [unwired: 1 in, 1 out]
          }
          event "FIND FCS FILE": Value Change {
            n148 = event-data() -> ()  [unwired: 1 in, 1 out]
            n149 = Enqueue Element(queue=w571, element=mm_states."FIND FCS FILE ", error in (no error)=w564) -> (queue out=w570:refnum<queue>, error out=w565:errorcluster)  [unwired: 1 in, 1 out]
          }
          event "START EXPERIMENT": Value Change {
            n150 = event-data() -> ()  [unwired: 1 in, 2 out]
            n151 = Enqueue Element(queue=w583, element=mm_states."START EXPERIMENT", error in (no error)=w581) -> (queue out=w582:refnum<queue>, error out=w580:errorcluster)  [unwired: 1 in, 1 out]
          }
        }
      }
      frame "INITIALIZE INSTRUMENT" {
        n152 = Send Notification(notification=robotics_states."BUSY", notifier=w611, error in (no error)=w610) -> (notifier out=w604:refnum<notifier>, error out=w609:errorcluster)
        n153 = Send Notification(notification=w587, notifier=w616, error in (no error)=w609) -> (notifier out=w612:refnum<notifier>, error out=w615:errorcluster)
        n154 = Enqueue Element(queue=w619, element=hts_message."INITIALIZE", error in (no error)=w615) -> (queue out=w617:refnum<queue>, error out=w597:errorcluster)  [unwired: 1 in, 1 out]
        n155 = Get Notifier Status(notifier=w598, error in (no error)=w597) -> (notifier out=w593:refnum<notifier>, current notification=w596:T2, error out=w595:errorcluster)  [unwired: 2 out]
        n156 = Unbundle By Name(w596) -> ("USE LIGHTS?"=w591:bool)
        n157 = case shown="True" w591 {
          tunnel: w600 -> [w621 w626]
          tunnel: [w621 w624] -> w599
          tunnel: w595 -> [w620 w623]
          tunnel: [w620 w622] -> w594
          frame False {
          }
          frame True {
            n158 = Enqueue Element(queue=w626, element=led_mm."INITALIZE", error in (no error)=w623) -> (queue out=w624:refnum<queue>, error out=w622:errorcluster)  [unwired: 1 in, 1 out]
          }
        }
        n159 = Enqueue Element(queue=w607, element=data_message."INITIALIZE", error in (no error)=w594) -> (queue out=w606:refnum<queue>, error out=w584:errorcluster)  [unwired: 1 in, 1 out]
        n160 = call "set_sample_number.vi"("ERROR IN"=w584, "EXP SETTINGS"=w585) -> ("error out"=w589:errorcluster, "EXP SETTINGS UPDATED"=w588:refnum<notifier>)  [unwired: 8 in]
        n161 = call "wait_on_robots.vi"("error in (no error)"=w589, "Notifier in"=w604) -> ("error out"=w590:errorcluster, "Notifier out"=w603:refnum<notifier>)  [unwired: 8 in]
        n162 = Enqueue Element(queue=w614, element=mm_states."WAIT FOR COMMAND", error in (no error)=w590) -> (queue out=w613:refnum<queue>, error out=w592:errorcluster)  [unwired: 1 in, 1 out]
      }
      frame "FIND FCS FILE " {
        n163 = Send Notification(notification=w627, notifier=w657, error in (no error)=w656) -> (notifier out=w655:refnum<notifier>, error out=w651:errorcluster)
        n164 = Get Notifier Status(notifier=w652, error in (no error)=w651) -> (notifier out=w632:refnum<notifier>, current notification=w650:T2, error out=w648:errorcluster)  [unwired: 2 out]
        n165 = Unbundle By Name(w650) -> ("FACS DIVA DIRECTORY"=w649:path)
        n166 = call "find_newest_file.vi"("error in"=w648, "Directory Path to Start the Search"=w649) -> ("error out"=w647:errorcluster, "Most Recent File Path"=w629:path)  [unwired: 6 in, 1 out]
        "?" <- w629
        n167 = call "fcs_read.vi"("error in (no error)"=w647, "Path"=w629) -> ("error out"=w645:errorcluster, "byte offset"=w643:i64)  [unwired: 6 in, 2 out]
        n168 = Get Notifier Status(notifier=w646, error in (no error)=w645) -> (notifier out=w642:refnum<notifier>, current notification=w644:T12, error out=w641:errorcluster)  [unwired: 2 out]
        n169 = Bundle By Name(cluster=w644, "fcs file byte offset"=w643, "FCS FILE PATH"=w629) -> (w639:T12)
        n170 = Send Notification(notification=w639, notifier=w642, error in (no error)=w641) -> (notifier out=w640:refnum<notifier>, error out=w636:errorcluster)
        n171 = Enqueue Element(queue=w638, element=mm_states."WAIT FOR COMMAND", error in (no error)=w636) -> (queue out=w637:refnum<queue>, error out=w635:errorcluster)  [unwired: 1 in, 1 out]
      }
      frame "WAIT TO SAMPLE " {
        n172 = Send Notification(notification=w663, notifier=w686, error in (no error)=w685) -> (notifier out=w681:refnum<notifier>, error out=w659:errorcluster)
        n173 = call "set_sample_number.vi"("ERROR IN"=w659, "EXP SETTINGS"=w658) -> ("error out"=w678:errorcluster, "EXP SETTINGS UPDATED"=w677:refnum<notifier>)  [unwired: 8 in]
        n174 = call "set_experiment_state.vi"("error in (no error)"=w678, "GLOBAL SETTINGS IN"=w683, "EXPERIMENT SETTINGS IN"=w677) -> ("error out"=w675:errorcluster, "GLOBAL SETTINGS OUT"=w674:refnum<notifier>, "EXPERIMENT SETTINGS OUT"=w676:refnum<notifier>)  [unwired: 6 in]
        n175 = Get Notifier Status(notifier=w674) -> (notifier out=w660:refnum<notifier>, current notification=w673:T2)  [unwired: 1 in, 3 out]
        n176 = Unbundle By Name(w673) -> ("SECONDS BETWEEN SAMPLING"=w672:dbl)
        n177 = while {
          tunnel: [w692] -> w668
          tunnel: [w691] -> w662
          tunnel: w676 -> [w690]
          tunnel: w675 -> [w689]
          tunnel: w672 -> [w687]
          tunnel: w671 -> [w688]
          stop <- w700 stop-if-true
          n178 = call "Elapsed Time3"("Time Target (s)"=w687, "Set Start Time (s)"=w688) -> ("Elapsed Time (s)"=w699:dbl, "Time has Elapsed"=w700:bool)  [unwired: 10 in, 6 out]
          n179 = Get Notifier Status(notifier=w690, error in (no error)=w689) -> (notifier out=w695:refnum<notifier>, current notification=w698:T12, error out=w694:errorcluster)  [unwired: 2 out]
          n180 = Subtract(x=w687, y=w699) -> (x-y=w697:dbl)
          n181 = Bundle By Name(cluster=w698, "TIME TILL SAMPLE"=w697) -> (w696:T12)
          n182 = Wait (ms)(milliseconds to wait=u32 500) -> ()  [unwired: 1 out]
          n183 = Send Notification(notification=w696, notifier=w695, error in (no error)=w694) -> (notifier out=w691:refnum<notifier>, error out=w692:errorcluster)
        }
        n184 = Enqueue Element(queue=w670, element=mm_states."TAKE SAMPLE ", error in (no error)=w668) -> (queue out=w669:refnum<queue>, error out=w667:errorcluster)  [unwired: 1 in, 1 out]
        n185 = call "update_exp_time.vi"("error in"=w667) -> ("error out"=w666:errorcluster, "double precision float"=w665:dbl)  [unwired: 9 in]
      }
      frame "TAKE SAMPLE " {
        n186 = Send Notification(notification=w707, notifier=w776, error in (no error)=w770) -> (notifier out=w773:refnum<notifier>, error out=w742:errorcluster)
        n187 = Send Notification(notification=robotics_states."BUSY", notifier=w743, error in (no error)=w742) -> (notifier out=w725:refnum<notifier>, error out=w724:errorcluster)
        n188 = Enqueue Element(queue=w746, element=data_message."THROW AWAY DATA", error in (no error)=w724) -> (queue out=w745:refnum<queue>, error out=w723:errorcluster)  [unwired: 1 in, 1 out]
        n189 = call "increment_sample_number.vi"("error in"=w723, "EXPERIMENT SETTINGS IN"=w771) -> ("error out"=w726:errorcluster, "EXPERIMENT SETTINGS OUT"=w716:refnum<notifier>)  [unwired: 8 in]
        n190 = call "wait_on_robots.vi"("error in (no error)"=w726, "Notifier in"=w725) -> ("error out"=w761:errorcluster, "Notifier out"=w759:refnum<notifier>)  [unwired: 8 in]
        n191 = Send Notification(notification=robotics_states."BUSY", notifier=w759, error in (no error)=w761) -> (notifier out=w758:refnum<notifier>, error out=w760:errorcluster)
        n192 = Enqueue Element(queue=w727, element=hts_message."SAMPLE REACTOR", error in (no error)=w760) -> (queue out=w740:refnum<queue>, error out=w774:errorcluster)  [unwired: 1 in, 1 out]
        n193 = call "wait_on_robots.vi"("error in (no error)"=w774, "Notifier in"=w758) -> ("error out"=w764:errorcluster, "Notifier out"=w765:refnum<notifier>)  [unwired: 8 in]
        n194 = Send Notification(notification=robotics_states."BUSY", notifier=w765, error in (no error)=w764) -> (notifier out=w757:refnum<notifier>, error out=w762:errorcluster)
        n195 = Enqueue Element(queue=w745, element=data_message."UPDATE DATA", error in (no error)=w762) -> (queue out=w753:refnum<queue>, error out=w751:errorcluster)  [unwired: 1 in, 1 out]
        n196 = Enqueue Element(queue=w753, element=data_message."ANALYZE DATA", error in (no error)=w751) -> (queue out=w752:refnum<queue>, error out=w750:errorcluster)  [unwired: 1 in, 1 out]
        n197 = Enqueue Element(queue=w752, element=data_message."SAVE DATA", error in (no error)=w750) -> (queue out=w722:refnum<queue>, error out=w749:errorcluster)  [unwired: 1 in, 1 out]
        n198 = call "wait_on_robots.vi"("error in (no error)"=w749, "Notifier in"=w757) -> ("error out"=w755:errorcluster, "Notifier out"=w756:refnum<notifier>)  [unwired: 8 in]
        n199 = Send Notification(notification=robotics_states."BUSY", notifier=w756, error in (no error)=w755) -> (notifier out=w721:refnum<notifier>, error out=w739:errorcluster)
        n200 = Enqueue Element(queue=w740, element=hts_message."CLEAR LINES", error in (no error)=w739) -> (queue out=w737:refnum<queue>, error out=w720:errorcluster)  [unwired: 1 in, 1 out]
        n201 = call "wait_on_robots.vi"("error in (no error)"=w720, "Notifier in"=w721) -> ("error out"=w734:errorcluster, "Notifier out"=w732:refnum<notifier>)  [unwired: 8 in]
        n202 = Send Notification(notification=robotics_states."BUSY", notifier=w732, error in (no error)=w734) -> (notifier out=w729:refnum<notifier>, error out=w733:errorcluster)
        n203 = Enqueue Element(queue=w737, element=hts_message."MOVE TO NEXT", error in (no error)=w733) -> (queue out=w736:refnum<queue>, error out=w730:errorcluster)  [unwired: 1 in, 1 out]
        n204 = call "wait_on_robots.vi"("error in (no error)"=w730, "Notifier in"=w729) -> ("error out"=w714:errorcluster, "Notifier out"=w728:refnum<notifier>)  [unwired: 8 in]
        n205 = Get Notifier Status(notifier=w716, error in (no error)=w714) -> (notifier out=w715:refnum<notifier>, current notification=w719:T12, error out=w718:errorcluster)  [unwired: 2 out]
        n206 = Get Notifier Status(notifier=w713, error in (no error)=w718) -> (notifier out=w708:refnum<notifier>, current notification=w717:T2, error out=w710:errorcluster)  [unwired: 2 out]
        n207 = Unbundle By Name(w717) -> ("# REACTORS"=w705:u32, "OUTGROWTH TIME POINTS"=w702:dbl)
        n208 = Unbundle By Name(w719) -> ("SAMPLE #"=w706:i32, "TIME POINT"=w703:i32)
        n209 = Equal?(x=w706, y=w705) -> (x = y?=w704:bool)
        n210 = Equal?(x=w703, y=w702) -> (x = y?=w701:bool)
        n211 = case shown="True" w704 {
          tunnel: [w780 w786] -> w712
          tunnel: w711 -> [w781 w785]
          tunnel: w710 -> [w779 w784]
          tunnel: [w778 w783] -> w709
          tunnel: w701 -> [_ w782]
          frame False {
            n212 = Enqueue Element(queue=w781, element=mm_states."TAKE SAMPLE ", error in (no error)=w779) -> (queue out=w780:refnum<queue>, error out=w778:errorcluster)  [unwired: 1 in, 1 out]
          }
          frame True {
            n213 = case shown="True" w782 {
              tunnel: [w791 w795] -> w786
              tunnel: w785 -> [w790 w796]
              tunnel: w784 -> [w789 w793]
              tunnel: [w788 w794] -> w783
              frame False {
                n214 = Enqueue Element(queue=w790, element=mm_states."WAIT TO SAMPLE ", error in (no error)=w789) -> (queue out=w791:refnum<queue>, error out=w788:errorcluster)  [unwired: 1 in, 1 out]
              }
              frame True {
                n215 = Enqueue Element(queue=w796, element=mm_states."DILUTE", error in (no error)=w793) -> (queue out=w795:refnum<queue>, error out=w794:errorcluster)  [unwired: 1 in, 1 out]
              }
            }
          }
        }
      }
      frame "DILUTE" {
        n216 = Send Notification(notification=w803, notifier=w802, error in (no error)=w805) -> (notifier out=w801:refnum<notifier>, error out=w804:errorcluster)
        n217 = Send Notification(notification=robotics_states."BUSY", notifier=w819, error in (no error)=w804) -> (notifier out=w816:refnum<notifier>, error out=w818:errorcluster)
        n218 = Enqueue Element(queue=w817, element=hts_message."DILUTE AND INDUCE", error in (no error)=w818) -> (queue out=w798:refnum<queue>, error out=w815:errorcluster)  [unwired: 1 in, 1 out]
        n219 = call "wait_on_robots.vi"("error in (no error)"=w815, "Notifier in"=w816) -> ("error out"=w800:errorcluster, "Notifier out"=w799:refnum<notifier>)  [unwired: 8 in]
        n220 = Enqueue Element(queue=w810, element=mm_states."WAIT TO SAMPLE ", error in (no error)=w800) -> (queue out=w808:refnum<queue>, error out=w809:errorcluster)  [unwired: 1 in, 1 out]
      }
      frame "EXIT" {
        n221 = Send Notification(notification=w822, notifier=w836, error in (no error)=w835) -> (notifier out=w824:refnum<notifier>, error out=w834:errorcluster)
        n222 = Enqueue Element(queue=w838, element=data_message."SHUTDOWN", error in (no error)=w834) -> (queue out=w837:refnum<queue>, error out=w833:errorcluster)  [unwired: 1 in, 1 out]
        n223 = Enqueue Element(queue=w831, element=hts_message."SHUTDOWN", error in (no error)=w833) -> (queue out=w830:refnum<queue>, error out=w832:errorcluster)  [unwired: 1 in, 1 out]
        n224 = Enqueue Element(queue=w829, element=led_mm."SHUTDOWN", error in (no error)=w832) -> (queue out=w828:refnum<queue>, error out=w823:errorcluster)  [unwired: 1 in, 1 out]
      }
      frame "START EXPERIMENT" {
        n225 = Send Notification(notification=w858, notifier=w880, error in (no error)=w879) -> (notifier out=w850:refnum<notifier>, error out=w856:errorcluster)
        n226 = Get Notifier Status(notifier=w857, error in (no error)=w856) -> (notifier out=w847:refnum<notifier>, current notification=w855:T2, error out=w854:errorcluster)  [unwired: 2 out]
        n227 = Unbundle By Name(w855) -> ("REACTORS TO USE"=w853:u32[])
        n228 = Get Date/Time In Seconds() -> (seconds since 1Jan1904=w868:timestamp)
        "?" <- w868
        n229 = Get Notifier Status(notifier=w878, error in (no error)=w854) -> (notifier out=w875:refnum<notifier>, current notification=w877:T12, error out=w874:errorcluster)  [unwired: 2 out]
        n230 = Index Array(array=w853, index=0) -> (element=w851:u32)
        n231 = Bundle By Name(cluster=w877, "CURRENT VALVE"=w851, "START TIME"=w868) -> (w873:T12)
        n232 = Send Notification(notification=w873, notifier=w875, error in (no error)=w874) -> (notifier out=w862:refnum<notifier>, error out=w864:errorcluster)
        n233 = call "update_exp_state.vi"("ERROR IN"=w864, "NEW STATE"=experiment_states."OUTGROWTH", "EXP SETTINGS"=w862) -> ("ERROR OUT"=w863:errorcluster, "EXP SETTINGS UPDATED"=w861:refnum<notifier>)  [unwired: 7 in]
        n234 = Enqueue Element(queue=w876, element=mm_states."TAKE SAMPLE ", error in (no error)=w863) -> (queue out=w872:refnum<queue>, error out=w865:errorcluster)  [unwired: 1 in, 1 out]
        n235 = call "update_exp_time.vi"("error in"=w865) -> ("error out"=w846:errorcluster, "double precision float"=w867:dbl)  [unwired: 9 in]
        n236 = call "start_leds.vi"("ERROR IN"=w846, "notifier out"=w847, "LED THREAD"=w849) -> ("error out"=w845:errorcluster, "LED THREAD OUT"=w848:refnum<queue>)  [unwired: 7 in]
      }
    }
    n237 = Or(x=w464, y=FALSE) -> (x .or. y?=w463:bool)
  }
  n238 = Release Queue(queue=w67, error in (no error)=w66) -> ()  [unwired: 4 out]
  n239 = Release Notifier(notifier=w48) -> ()  [unwired: 2 in, 3 out]
  n240 = Release Notifier(notifier=w68) -> ()  [unwired: 2 in, 3 out]
  n241 = Release Notifier(notifier=w64) -> ()  [unwired: 2 in, 3 out]
  n242 = Release Notifier(notifier=w47) -> ()  [unwired: 2 in, 3 out]
  n243 = Release Notifier(notifier=w29) -> ()  [unwired: 2 in, 3 out]
  n244 = Release Queue(queue=w83, error in (no error)=w70) -> ()  [unwired: 4 out]
  n245 = Release Notifier(notifier=w51) -> ()  [unwired: 2 in, 3 out]
  n246 = Release Notifier(notifier=w73) -> ()  [unwired: 2 in, 3 out]
  n247 = Release Notifier(notifier=w71) -> ()  [unwired: 2 in, 3 out]
  n248 = Release Notifier(notifier=w31) -> ()  [unwired: 2 in, 3 out]
  n249 = Release Notifier(notifier=w52) -> ()  [unwired: 2 in, 3 out]
  n250 = call "leds_queue.vi"() -> ("queue out"=w45:refnum<queue>)  [unwired: 10 in, 1 out]
  n251 = call "strobe_timer.vi"() -> ("error out"=w43:errorcluster, "notifier out"=w44:refnum<notifier>)  [unwired: 10 in]
  n252 = call "global_state_notifier.vi"() -> ("GLOBAL STATE"=w13:refnum<notifier>)  [unwired: 10 in, 1 out]
  n253 = call "settings_notifier.vi"() -> ("GLOBAL SETTINGS"=w24:refnum<notifier>)  [unwired: 10 in, 1 out]
  n254 = call "reactors_notifier.vi"() -> ("Notifier out"=w25:refnum<notifier>)  [unwired: 10 in, 1 out]
  n255 = call "experiment_settings.vi"() -> ("Notifier out"=w35:refnum<notifier>)  [unwired: 10 in, 1 out]
  n256 = call "global_state_notifier.vi"() -> ("error out"=w23:errorcluster, "GLOBAL STATE"=w37:refnum<notifier>)  [unwired: 10 in]
  n257 = call "robotics_state.vi"() -> ("Notifier out"=w36:refnum<notifier>)  [unwired: 10 in, 1 out]
  n258 = call "machine_thread_states.vi"() -> ("Notifier out"=w26:refnum<notifier>)  [unwired: 10 in, 1 out]
  n259 = Release Queue(queue=w59, error in (no error)=w60) -> ()  [unwired: 4 out]
  n260 = Release Notifier(notifier=w55) -> ()  [unwired: 2 in, 3 out]
  n261 = Release Notifier(notifier=w56) -> ()  [unwired: 2 in, 3 out]
  n262 = Release Notifier(notifier=w53) -> ()  [unwired: 2 in, 3 out]
  n263 = Release Notifier(notifier=w33) -> ()  [unwired: 2 in, 3 out]
  n264 = Release Notifier(notifier=w27) -> ()  [unwired: 2 in, 3 out]
  n265 = Wait on Notification(notifier=w44, error in (no error)=w43) -> (notifier out=w41:refnum<notifier>, error out=w9:errorcluster)  [unwired: 2 in, 2 out]
  n266 = call "update_exp_time.vi"("error in"=w9) -> ("error out"=w8:errorcluster, "double precision float"=w10:dbl)  [unwired: 9 in]
  n267 = Get Notifier Status(notifier=w24, error in (no error)=w8) -> (notifier out=w38:refnum<notifier>, current notification=w39:T2, error out=w40:errorcluster)  [unwired: 2 out]
  n268 = while {
    tunnel: w37 -> [w897]
    tunnel: w36 -> [w899]
    tunnel: w35 -> [w900]
    tunnel: w26 -> [w898]
    tunnel: w25 -> [w901]
    tunnel: [w892] -> w22
    tunnel: [w891] -> w21
    tunnel: [w890] -> w20
    tunnel: [w889] -> w19
    shift-right: [w888] -> w18
    shift-left: w23 -> [w894]
    tunnel: [w887] -> w17
    stop <- w896 stop-if-true
    n269 = Get Notifier Status(notifier=w897, error in (no error)=w894) -> (notifier out=w895:refnum<notifier>, current notification=w882:T1, error out=w893:errorcluster)  [unwired: 2 out]
    "GLOBAL STATE" <- w882
    n270 = Equal?(x=w882, y=mm_states."EXIT") -> (x = y?=w896:bool)
    n271 = event shown="[0] Timeout" {
      selector: _ -> [_ _ _ _]
      dyn-events: _ -> [_ _ _ _]
      timeout: 1000 -> [_ _ _ _]
      tunnel: w901 -> [w912 w929 w962 w984]
      tunnel: w900 -> [w922 w939 w957 w993]
      tunnel: w899 -> [w920 w937 w945 w967]
      tunnel: w898 -> [w917 w934 w943 w969]
      tunnel: w895 -> [w919 w936 w958 w995]
      tunnel: [w919 w936 w958 w995] -> w890
      tunnel: [w918 w935 w944 w966] -> w889
      tunnel: w893 -> [w916 w933 w956 w992]
      tunnel: [w913 w930 w952 w985] -> w888
      tunnel: [w912 w929 w959 w983] -> w892
      tunnel: [w911 w928 w947 w964] -> w891
      tunnel: [w910 w927 w942 w968] -> w887
      tunnel: [w909 w926 w951 w990] -> w886
      tunnel: [w908 w925 w949 w988] -> w884
      tunnel: [w907 w924 w950 w989] -> w885
      tunnel: [w906 w923 w940 w963] -> w883
      event Timeout {
        n272 = event-data() -> ()  [unwired: 1 in, 3 out]
        n273 = Get Notifier Status(notifier=w922, error in (no error)=w916) -> (notifier out=w911:refnum<notifier>, current notification=w921:T12, error out=w915:errorcluster)  [unwired: 2 out]
        n274 = Get Notifier Status(notifier=w920, error in (no error)=w915) -> (notifier out=w918:refnum<notifier>, current notification=w909:T11, error out=w914:errorcluster)  [unwired: 2 out]
        n275 = Get Notifier Status(notifier=w917, error in (no error)=w914) -> (notifier out=w910:refnum<notifier>, error out=w913:errorcluster)  [unwired: 3 out]
        n276 = Unbundle By Name(w921) -> ("STATE"=→"EXPERIMENT STATE":T3, "TIME POINT"=w906:i32, "CURRENT VALVE"=w907:u32, "SAMPLE #"=w908:i32, "TIME TILL SAMPLE"=→"TIME TILL SAMPLE":dbl, "DILUTION  TABLE"=→"DILUTION  TABLE":dbl[][])
      }
      event "UPDATE STATES": Value Change {
        n277 = event-data() -> ()  [unwired: 1 in, 6 out]
        n278 = Get Notifier Status(notifier=w939, error in (no error)=w933) -> (notifier out=w928:refnum<notifier>, current notification=w938:T12, error out=w932:errorcluster)  [unwired: 2 out]
        n279 = Get Notifier Status(notifier=w937, error in (no error)=w932) -> (notifier out=w935:refnum<notifier>, current notification=w926:T11, error out=w931:errorcluster)  [unwired: 2 out]
        n280 = Get Notifier Status(notifier=w934, error in (no error)=w931) -> (notifier out=w927:refnum<notifier>, error out=w930:errorcluster)  [unwired: 3 out]
        n281 = Unbundle By Name(w938) -> ("TIME POINT"=w923:i32, "CURRENT VALVE"=w924:u32, "SAMPLE #"=w925:i32)  [unwired: 2 out]
      }
      event "SHOW REACTOR": Value Change {
        n282 = event-data() -> ()  [unwired: 1 in, 2 out]
        n283 = Get Notifier Status(notifier=w957, error in (no error)=w956) -> (notifier out=w947:refnum<notifier>, current notification=w948:T12, error out=w955:errorcluster)  [unwired: 2 out]
        n284 = Get Notifier Status(notifier=w962, error in (no error)=w955) -> (notifier out=w959:refnum<notifier>, current notification=w961:T14, error out=w954:errorcluster)  [unwired: 2 out]
        n285 = Decrement(x="REACTOR #") -> (x-1=w946:i32)
        n286 = Get Notifier Status(notifier=w945, error in (no error)=w954) -> (notifier out=w944:refnum<notifier>, current notification=w951:T11, error out=w953:errorcluster)  [unwired: 2 out]
        n287 = Index Array(array=w961, index=w946) -> (element=→"REACTOR":T5)
        n288 = Get Notifier Status(notifier=w943, error in (no error)=w953) -> (notifier out=w942:refnum<notifier>, error out=w952:errorcluster)  [unwired: 3 out]
        n289 = Unbundle By Name(w948) -> ("TIME POINT"=w940:i32, "CURRENT VALVE"=w950:u32, "SAMPLE #"=w949:i32)  [unwired: 2 out]
      }
      event "GRAPH DATA": Value Change {
        n290 = event-data() -> ()  [unwired: 1 in, 2 out]
        n291 = Get Notifier Status(notifier=w993, error in (no error)=w992) -> (notifier out=w965:refnum<notifier>, error out=w987:errorcluster)  [unwired: 3 out]
        n292 = Get Notifier Status(notifier=w967, error in (no error)=w987) -> (notifier out=w966:refnum<notifier>, current notification=w990:T11, error out=w991:errorcluster)  [unwired: 2 out]
        n293 = Get Notifier Status(notifier=w969, error in (no error)=w991) -> (notifier out=w968:refnum<notifier>, current notification=w994:cluster{T6, "COMMAND":T8, T7}, error out=w976:errorcluster)  [unwired: 2 out]
        n294 = property on="LOG FITC/SSC" class="WFChart (strict)"(error in=w976, "History Data"=dbl[] []) -> (error out=w975:errorcluster)  [unwired: 1 in, 1 out]
        n295 = property on="LOG (X/Y)" class="WFGraph (strict)"(error in=w975, "Value"=dynamicdata [] ("LOG (X/Y)")) -> (error out=w974:errorcluster)  [unwired: 1 in, 1 out]
        n296 = Unbundle(w994) -> ()  [unwired: 3 out]
        n297 = property on="Y VERSUS X" class="XYGraph (strict)"(error in=w974, "Value"=T10 {"LAST MEASUREMENT"=[], "LAST MEASUREMENT"=[]} ("Y VERSUS X")) -> (error out=w973:errorcluster)  [unwired: 1 in, 1 out]
        n298 = call "graph_data.vi"("Notifier in"=w984, "X"="X", "Y"="Y", "Reactor to display"="Reactor to Graph") -> ("Notifier in 2"=w983:refnum<notifier>, "Cluster"=→"Y VERSUS X":T16, "Histogram"=→"LOG (X/Y)":dynamicdata, "SUMMARY STATS GRAPH"=→"LOG FITC/SSC":dbl[])  [unwired: 3 in]
        n299 = Get Notifier Status(notifier=w965, error in (no error)=w973) -> (notifier out=w964:refnum<notifier>, current notification=w986:T12, error out=w985:errorcluster)  [unwired: 2 out]
        n300 = Unbundle By Name(w986) -> ("TIME POINT"=w963:i32, "CURRENT VALVE"=w989:u32, "SAMPLE #"=w988:i32)
      }
    }
    "ROBOTICS READY?" <- w886
    "CURRENT VALVE" <- w885
    "SAMPLE #" <- w884
    "TIME POINT" <- w883
  }
  n301 = while {
    tunnel: w41 -> [w1013]
    tunnel: w45 -> [w1011]
    tunnel: w39 -> [w1015]
    tunnel: w38 -> [w1012]
    tunnel: [w1012] -> w42
    shift-right: [w997] -> w14
    shift-left: w40 -> [w1009]
    tunnel: w13 -> [w1010]
    tunnel: [w1007] -> w12
    shift-right: [w996] -> _
    shift-left: w10 -> [w1002]
    tunnel: [w999] -> w7
    tunnel: [w998] -> w6
    stop <- w1004 stop-if-true
    n302 = Get Notifier Status(notifier=w1010, error in (no error)=w1009) -> (notifier out=w1007:refnum<notifier>, current notification=w1005:T1, error out=w1008:errorcluster)  [unwired: 2 out]
    n303 = Unbundle By Name(w1015) -> ("PULSE PERIOD"=w1014:i32)
    n304 = Equal?(x=w1005, y=ps_states."EXIT" ("latest notification")) -> (x = y?=w1004:bool)
    n305 = flat-sequence {
      tunnel: w1008 -> [w1021]
      tunnel: w1014 -> [w1017]
      tunnel: w1013 -> [w1018]
      tunnel: w1011 -> [w1020]
      tunnel: [w1020] -> w1003
      tunnel: w1002 -> [w1019]
      tunnel: [w1018] -> w1001
      tunnel: [w1016] -> w1000
      tunnel: w1003 -> [w1030]
      tunnel: w1001 -> [w1037]
      tunnel: [w1037] -> w998
      tunnel: w1000 -> [w1036]
      tunnel: [w1034] -> w999
      tunnel: [w1032] -> w997
      tunnel: [w1031] -> w996
      frame #0 {
        n306 = while {
          tunnel: w1021 -> [w1029]
          tunnel: w1019 -> [w1028]
          tunnel: w1017 -> [w1023]
          tunnel: [w1027] -> w1016
          stop <- w1025 stop-if-true
          n307 = call "Elapsed Time2"("Time Target (s)"=w1023, "error in (no error)"=w1029, "Set Start Time (s)"=w1028) -> ("Elapsed Time (s)"=w1024:dbl, "Time has Elapsed"=w1025:bool, "error out"=w1027:errorcluster)  [unwired: 9 in, 5 out]
          n308 = Wait (ms)(milliseconds to wait=u32 500) -> ()  [unwired: 1 out]
          n309 = Subtract(x=w1023, y=w1024) -> (x-y=→"TIME TILL STROBE":dbl)
        }
      }
      frame #1 {
        n310 = Enqueue Element(queue=w1030, element=led_mm."STROBE", error in (no error)=w1036) -> (queue out=w1034:refnum<queue>, error out=w1033:errorcluster)  [unwired: 1 in, 1 out]
        n311 = call "update_exp_time.vi"("error in"=w1033) -> ("error out"=w1032:errorcluster, "double precision float"=w1031:dbl)  [unwired: 9 in]
      }
    }
  }
  n312 = Release Queue(queue=w7) -> ()  [unwired: 1 in, 4 out]
  n313 = Release Notifier(notifier=w6) -> ()  [unwired: 2 in, 3 out]
  n314 = Release Notifier(notifier=w12) -> ()  [unwired: 2 in, 3 out]
  n315 = Release Notifier(notifier=w42, error in (no error)=w14) -> ()  [unwired: 1 in, 3 out]
  n316 = Release Notifier(notifier=w22) -> ()  [unwired: 2 in, 3 out]
  n317 = Release Notifier(notifier=w21) -> ()  [unwired: 2 in, 3 out]
  n318 = Release Notifier(notifier=w20, error in (no error)=w18) -> ()  [unwired: 1 in, 3 out]
  n319 = Release Notifier(notifier=w19) -> ()  [unwired: 2 in, 3 out]
  n320 = Release Notifier(notifier=w17) -> ()  [unwired: 2 in, 3 out]
  n321 = Release Queue(queue=w96) -> ()  [unwired: 1 in, 4 out]
  n322 = Release Queue(queue=w95) -> ()  [unwired: 1 in, 4 out]
  n323 = Release Queue(queue=w94) -> ()  [unwired: 1 in, 4 out]
  n324 = Release Notifier(notifier=w63) -> ()  [unwired: 2 in, 3 out]
  n325 = Release Notifier(notifier=w50) -> ()  [unwired: 2 in, 3 out]
  n326 = Release Notifier(notifier=w92) -> ()  [unwired: 2 in, 3 out]
  n327 = Release Notifier(notifier=w74) -> ()  [unwired: 2 in, 3 out]
  n328 = Release Queue(queue=w91, error in (no error)=w86) -> ()  [unwired: 4 out]
